vi "PRISM_RasterScan_BSC202(T-Dimension_Added).vi"() -> ()   [LabVIEW 2022 SP3]
uses:
  C:/Users/ulate/Documents/mnOP/mnOPSuite-main/PRISM/Thorlabs.MotionControl.Controls.dll
  mnOPSuite-main/PRISM/Thorlabs.MotionControl.Controls.dll
  C:/Users/ulate/Documents/mnOP/mnOPSuite-main/PRISM/Thorlabs.MotionControl.KCube.StepperMotorCLI.dll
  mnOPSuite-main/PRISM/Thorlabs.MotionControl.KCube.StepperMotorCLI.dll
  <vilib>/Analysis/NI_AALBase.lvlib
  <vilib>/Analysis/baseanly.llb/Mean (DBL).vi
  C:/Users/ulate/Documents/mnOP/mnOPSuite-main/PRISM/Thorlabs.MotionControl.Benchtop.StepperMotorCLI.dll
  mnOPSuite-main/PRISM/Thorlabs.MotionControl.Benchtop.StepperMotorCLI.dll
  mnOPSuite-main/PRISM/Control_PRISMRasterScan_ActivityLoop.ctl
  mnOPSuite-main/PRISM/Control_LineScanCounterAE.ctl
  mnOPSuite-main/PRISM/Control_PRISMRasterScan_ProtocolsLoop.ctl
  ActionEngineEnum.ctl
panel:
  in  "t Action":T1=enum."Done"
  out "t - Current Position (mm)":dbl
  in  "t Motor Settings":T2={"Step Size (mm)"=10.0, "Initial Position"=0.0, "Move Absolute/Relative Position"=0.0, "Step Delay (ms)"=0, "Velocity (mm/s)"=1.5, "Acceleration (mm/s^2)"=1.0} {"Step Size (mm)" min=0.00046 format="%.8f"}
  out "t error out":errorcluster
  in  "KCubeStepperControl t":refnum<k24>(container)
  in  "SerialNumber t":string="26004283"
  in  "Update origin":bool
  out "Protocol status":string="Ready for protocol!"
  in  "Protocols":T3(tab)=enum."Saved Positions"
  in  "Target coordinate":T4={"X coord (mm)"=13.679193173363094, "Y coord (mm)"=17.37439041210012, "Z coord (mm)"=19.037080609490427, "t coord (mm)"=0.0}
  in  "Move to target":bool
  out "Origin coordinate":T4={"X coord (mm)"=13.208955078125, "Y coord (mm)"=17.107802734375, "Z coord (mm)"=19.036842575356477, "t coord (mm)"=0.0}
  in  "Update target":bool
  in  "Move to origin":bool
  in  "Stored positions":T5(array[cluster])=[{"X coord (mm)"=15.5859716796875, "Y coord (mm)"=15.71225830078125, "Z coord (mm)"=19.053150660079638, "t coord (mm)"=0.0}, {"X coord (mm)"=13.679193173363094, "Y coord (mm)"=17.37439041210012, "Z coord (mm)"=19.037080609490427, "t coord (mm)"=0.0}, {"X coord (mm)"=9.08337158203125, "Y coord (mm)"=16.38648681640625, "Z coord (mm)"=19.027052048324006, "t coord (mm)"=0.0}]
  in  "Stored position names":string[](array[string])=["Gold", "Corner", "Shane region"]
  in  "Move to\nstored position":bool[](array[boolean])=[FALSE, FALSE, FALSE]
  in  "Store target\nposition to":bool[](array[boolean])=[FALSE, FALSE, FALSE]
  in  "Do Linescan":bool
  in  "Linescan points\n(relative x,y, microns)":dbl[][](array[numeric])=[[134.75975910445754, 60.57194852467012], [148.27256923926274, 62.20847306409274], [161.7853793740679, 63.84499760351537], [175.29818950887307, 65.48152214293799], [188.81099964367826, 67.11804668236061], [202.32380977848345, 68.75457122178324], [215.83661991328862, 70.39109576120586], [229.34943004809378, 72.02762030062848], [242.86224018289897, 73.66414484005111], [256.37505031770417, 75.30066937947373], [269.88786045250936, 76.93719391889636], [283.4006705873145, 78.57371845831898], [296.9134807221197, 80.2102429977416], [310.4262908569249, 81.84676753716423], [323.93910099173, 83.48329207658685], [337.4519111265352, 85.11981661600947], [350.9647212613404, 86.7563411554321], [364.4775313961456, 88.39286569485472], [377.9903415309508, 90.02939023427734], [391.5031516657559, 91.66591477369997]]
  in  "Linescan Accumulations":i32=11 min=1
  out "Current point":i32
  in  "Halt linescan":bool
  out "Current\naccumulation":i32=11
  in  "Generate\n# points\n(cursors 1&2)":bool
  in  "# Points":i32=20 min=2 max=100
  out "X stepper reference":refnum<k24>
  out "Y stepper reference":refnum<k24>
  in  "BenchtopStepperControl Y":refnum<k24>(container)
  in  "BenchtopStepperControl X":refnum<k24>(container)
  in  "Save Image":bool
  in  "Path to save image":path=path "D:/Dropbox/Data/PRISM/2023.05.23 - Brayden - CalibrationExperiment - 119nmGrating/5x5_9.1micron_monochromated.txt"
  in  "Move to cursor 1":bool
  in  "Auto-level phase":bool
  in  "Acquire":bool=TRUE
  in  "Settle Time Y":u32=500
  in  "2nd sideband factor":dbl=1.0
  in  "Settle Time X":u32=50
  in  "Py":dbl=-38.62030580980725 format="%_3f"
  in  "Px":dbl=63.19603906604226 format="%_3f"
  in  "1st sideband offset":dbl
  in  "Phase offset":dbl=-7.0317445278654365 format="%_3f"
  out "Phase":dbl[][](graph)=[[-0.022387540499821057, -2.058073888022488, -2.674115903484436, -2.9544519791983532, 0.9804648819298123, -0.21571753535931215, -1.8423350309242874, 1.9906478539609171, 2.5360374269275248, 2.656112089306447, 2.35744039612554, 1.9479416381106667, 1.3283110045095121, 0.8287830160341692, 0.0015003367418202629, -0.6042101212176902, -1.313129505955537, -2.0121744959565113, -2.8202574981697097, 2.82386999642312, 2.1056236578858005, 1.3825868635958933, 0.6516979802989589, -0.11705277330859332, -0.8663526332155058, -1.6488935896277255, -2.3898283311918362, -3.111747881862428, 2.354022610449217, 1.5981909201102198, 0.999097752100301, 0.11666767544505063, -0.6255420967363605, -1.344064191404911, -2.1083959373327517, -2.8419430799594565, 2.667384503490176, 1.9637011456735003, 1.2230875404057322, 0.49976096613480436, -0.19396741539229012, -1.0079793141447588, -1.7125457563331672, 3.059263850520008, 2.2710943441974045, 1.4829248378748154, 0.6947553315522121, -0.09341417477039116, -0.8815836810929802, -1.6697531874155693], [1.3628880674624408, -0.2630817845670128, -0.10980599380193556, -1.8345316004921504, -2.204085976347738, -0.14179729710883748, -1.2847852512940126, 2.9634721346216164, -2.815473176799607, -2.5973907021062708, -2.922850019605578, 2.9635213410531325, 2.4514727389564435, 1.8030287953244226, 1.0294730194139348, 0.4576671275139077, -0.27089481789525394, -0.9873673943323595, -1.7804895356639534, -2.3687185763918244, 3.14003843880214, 2.318275957039088, 1.737089720416126, 0.9172648738715132, -0.21566467221115104, -0.43893815331455244, -1.326304504354333, -2.0795219597874492, -2.916987708315201, 2.695457261994612, 2.0229011483410417, 1.171918489139145, 0.43802228817759925, -0.2801368330695517, -1.0396590157832648, -1.8024496700734431, -2.5632904960467613, 3.040122676411002, 2.346330734522372, 1.5444701977180024, 0.8263618586431427, 0.05569318859598482, -0.7071801917261205, -1.9342063736791282, -2.7223758800017315, 2.7726399208552657, 1.9844704145326624, 1.196300908210059, 0.40813140188747, -0.3800381044351191], [-3.066884103109013, 0.9729599729543059, 0.8274657505887806, -0.8521734837812724, -1.7610376922341295, 1.5856394803568339, 0.1268857548291482, -1.9691799992391434, -1.4484367584059132, -1.2676123760144762, -1.6187348635530725, -2.0480064271227203, -2.4007798568858334, 3.1161499915202935, 2.3473474349846413, 1.7619068509469216, 1.0789468726915707, 0.37216732621407544, -0.4886782343943743, -1.0358510858881864, -1.7925323857931978, -2.602999261436789, 2.9510587581194585, 2.2525199600469996, 1.2937303676530512, 0.8952483171540173, 0.010397577352765808, -0.704939673587532, -1.6342691150966857, -2.218708036019933, -2.9599800502081486, 2.5159200741562735, 1.8299109061018193, 1.0253986988047359, 0.25924289190646377, -0.49860314852613996, -1.2596561474008254, -1.9321767682116544, -2.6680856525186627, 2.866214678319018, 2.2123793056056122, 1.3704893856878222, 0.6060059677024476, -0.6444912906986779, -1.432660797021267, -2.2208303033438703, -3.0089998096664594, 2.4860159911905235, 1.6978464848679202, 0.9096769785453311], [-2.3965980652031176, 1.6227568075408518, 1.168964897317034, 1.4095316197290177, -2.8014709215206857, -2.2329707988617766, 2.1851936633849363, -0.34485343356651654, 0.14279525512465874, 0.3540126356171065, -0.044315893155403074, -0.482972843851039, -1.002422538441758, -1.6853905594341434, -2.440464573629015, -2.8891213399429176, 2.5877374062332876, 1.8374526951417636, 1.1486396741771507, 0.5247186443110969, -0.26949674326147743, -1.0848567982945525, -1.848210887792014, -2.5387805815220865, 3.0687085163085435, 2.3387104464322164, 1.54582113363902, 0.8121802971552299, -0.03824350311151292, -0.6778476179916666, -1.4224225887198862, -2.229314349052679, -2.944827148116417, 2.5193975756285525, 1.8168759345426118, 1.0311792634079424, 0.29301642014190676, -0.46532133283141874, -1.0983502953965996, -1.9054318285761838, -2.5634056945953745, 2.9290667229416556, 2.1510820393184567, 0.6452237922817723, -0.1429457140408168, -0.9311152203634201, -1.7192847266860092, -2.5074542330086125, 2.9875615678483705, 2.1993920615257814], [-1.6841800797532274, 1.81433573403317, 1.9335449128509756, 1.4953972828545172, -1.608539055796733, -0.7086282362391554, -2.492175019225904, 1.1043658709546023, 1.6255459898063904, 1.7377721010176739, 1.4066056895155938, 0.9893110706463943, 0.41623260003367335, -0.42402667241574044, -1.0364775587393407, -1.5391521320349355, -2.4206609441522122, -3.097728525000063, 2.5361868143635213, 1.9845966715424126, 1.1191387411501275, 0.24604967911620435, -0.4740298321180312, -1.2495097740212167, -1.8317788479276942, -2.5951763567334396, 2.937298895851523, 2.2443865176780733, 1.3180121470375852, 0.5932561040055369, -0.03891982944377759, -0.8281018784912177, -1.4177150586273903, -2.2919076513566807, -3.069067654983254, 2.446145320515516, 1.7009132945316843, 0.8706102384085312, 0.2977063161632074, -0.4803340445821007, -1.1888387915909675, -1.9456314651204565, -2.84988979467969, 1.9349388752622367, 1.1467693689396334, 0.35859986261704435, -0.42956964370555895, -1.2177391500281622, -2.0059086563507513, -2.7940781626733404], [-0.8973343669603029, 2.123126138782993, 2.8199224507415517, 1.905484194967828, -1.127661496481934, 1.174155302549254, -0.8533196886458425, 2.6598834334499006, 3.075510546275801, -3.10785068992406, 2.7955257385388705, 2.412595201150511, 1.8555829163744129, 1.1888865219585476, 0.5176127773060646, -0.1418990848609507, -0.920191338355826, -1.5600168316567231, -2.293106731159032, -2.836949357060698, 2.5281579597586266, 1.8007761476738473, 1.0855407276800229, 0.27144007547231297, -0.36334755803092733, -1.1714381725212952, -1.9216266601785001, -2.6465573895732213, 2.8876005318127866, 2.1127905891614738, 1.3791718764432055, 0.5015637852025137, -0.08529276139088182, -0.8980377283577994, -1.672430623348692, -2.3824589331447292, 3.104730299921389, 2.4645905880971313, 1.72661821951014, 0.922796133288017, 0.19702009512686658, -0.5421983101135623, -1.2888533901549053, -3.058531348936903, 2.436484451920098, 1.6483149455974946, 0.8601454392749055, 0.0719759329523022, -0.7161935733703011, -1.5043630796928902], [0.08388963387707804, 2.906088721948243, 2.6850986349242767, 0.27512112222713636, 1.1091449624488927, 2.5073112355343996, 0.7899138334549409, -2.1604437613067216, -1.811580954875117, -1.7532620930163745, -2.0518609798455962, -2.406820073200329, -2.9886310634991364, 2.6116717182552023, 1.8510266765310348, 1.2843187293208533, 0.4296141672480793, -0.22785376121727374, -0.9773335792860802, -1.492074426042434, -2.33843645279439, 3.126300272992971, 2.3987147516140475, 1.592480069562761, 1.0353996771496732, 0.21793488873515088, -0.4725206147675465, -1.2331384498445779, -2.052011387265793, -2.7718324467228115, 2.8171907769568136, 2.0922645338624832, 1.2879170715464276, 0.43866550742682264, -0.27113986038910554, -0.9592680085289338, -1.785050188935319, -2.344856830069869, -3.124976762825561, 2.3015383661274385, 1.666433266139851, 0.8354098135605348, 0.12994388903859644, -1.7688162659564455, -2.5569857722790417, 2.9380300285779484, 2.1498605222553557, 1.3616910159327524, 0.5735215096101491, -0.21464799671243995], [0.7730064791060114, -2.2422916004447355, -2.7603924915974503, 2.43347466633578, 0.08731074224383217, -2.308316997016306, 2.393768121573377, -0.7118451463719238, -0.3355634717218221, -0.341494301675878, -0.6173869601886164, -1.024429550421761, -1.6166729606095078, -2.2341935145882683, -2.911480529054126, 2.7224483054582116, 1.981053415771921, 1.2218363391617988, 0.6523104836249072, -0.059507404315208845, -0.9535593178525446, -1.6193221075455906, -2.3700117432027543, -3.1250855773976536, 2.4788625057042744, 1.5463840538120408, 0.9800371354102033, 0.19579475094657184, -0.5653468704770397, -1.3707899976227438, -2.052383065739953, -2.789031304527679, 2.713926729646005, 1.8692635741312635, 1.1709183504774643, 0.45359994241800194, -0.3443418710311015, -0.9802643856205293, -1.765450941430231, -2.581249237757593, 3.043986042708198, 2.265111288961471, 1.5420804523152292, -0.47910118297598814, -1.2672706892985843, -2.0554401956211805, -2.8436097019437767, 2.651406098913206, 1.8632365925906136, 1.0750670862680245], [0.2580695237139876, 0.6828682232009009, -2.0469861827754645, 2.946288830382736, 0.6935475619157456, -0.10756103977141507, -2.2857382865566542, 0.712782643772337, 1.1093310428349588, 1.1774677065998338, 0.7947546112530475, 0.3567449711397579, -0.2272672897086636, -0.7640476232136955, -1.5475436693311009, -2.148207546509873, -2.8732833743547275, 2.614759429965167, 1.9901999575950011, 1.3305097400488837, 0.155054665233056, -0.2799398459732281, -1.129929015531875, -1.7955541373238404, -2.3900822532263497, 3.0472113011399973, 2.3715703347198698, 1.6539055221121153, 0.7409813253426805, 0.07315321432771427, -0.6342971726609861, -1.3299365984528642, -2.0538581044309687, -2.916252721124213, 2.5622245639023866, 1.8576744350770582, 1.068926198989402, 0.4247753644850647, -0.37687037047335536, -1.1670272987173398, -1.7851786584145728, -2.603830732259585, 2.904408054135054, 0.8106139000044621, 0.022444393681865904, -0.7657251126407303, -1.5538946189633265, -2.3420641252859298, -3.130233631608526, 2.3647821692484747], [-3.115997453644919, 1.3909049739370483, -1.9508788518699776, -2.9830523341856505, 1.6363109571985834, 1.2173345121005736, -0.739468648264018, 2.103685643131244, 2.5505355075887337, 2.5707732107446466, 2.268128255213327, 1.7210402472322528, 1.2308655811346911, 0.6085752294328506, -0.1483003340097877, -0.7464704859366584, -1.4736619725918327, -2.132855638872755, -2.9063750039330003, 2.728870665982347, 2.2285459060256656, 1.2752214884418969, 0.40971309866165306, -0.2857114181179359, -0.9826548217669391, -1.8061567137429009, -2.4775345698111977, 2.9629138369751384, 2.2654765680432583, 1.507411181145983, 0.7777850501704258, 0.07485373885175406, -0.6578077982824837, -1.4464199927970682, -2.2489490333640596, -2.981886614680178, 2.4773857903899454, 1.8533544801102124, 1.0099960800319217, 0.25794269886597476, -0.38849009668585666, -1.163266010818134, -1.961255983791105, 2.1003289829849194, 1.3121594766623232, 0.523989970339727, -0.26417953598286914, -1.0523490423054724, -1.8405185486280686, -2.6286880549506577], [-2.973824639667331, -0.3808371761856719, -1.2697167652686812, -2.250656583574277, 2.8690963540737027, 2.8392143717039797, 0.8135335245491242, -2.709993525842972, -2.3106513014105543, -2.3472060220939985, -2.5575537636549854, 3.120687882907709, 2.6305678861935364, 2.0085906949027024, 1.2420061608844648, 0.6335744611619436, -0.09758461693938791, -0.7620617457308008, -1.4573633096672136, -2.1472818673513068, -2.9396884225341697, 2.611867804818674, 1.738198702707928, 1.017938761103924, 0.40206618714671905, -0.3647565931770451, -1.1125631607993025, -1.829479741397277, -2.6132072700993483, 2.939980242492741, 2.1431631699713876, 1.4903147682332616, 0.7395956791538545, -0.09560326657526019, -0.8023186722421976, -1.55563412134617, -2.3724378835270095, -3.034613022697915, 2.4875320249892674, 1.7179354468544759, 1.0208687081664785, 0.2498819015875675, -0.5050262473460911, -2.8931412412142166, 2.6018745596427735, 1.8137050533201773, 1.025535546997581, 0.2373660406749778, -0.5508034656476184, -1.3389729719702075], [0.5200492600706852, 1.2630973959723146, -0.4740267800265876, -0.7403538003570418, -1.6536060683733167, -2.0800365358772215, 2.4503654239413013, -1.2585126799975002, -0.8877822370387727, -0.9313533566473948, -1.1973711148108261, -1.7177401303750703, -2.2263558951525066, -2.874595724811934, 2.643689238760323, 2.073831528075572, 1.3301628193342507, 0.6522957131674332, -0.03622715939361232, -0.7544934399100285, -1.5390794884192118, -2.17326521527799, -2.999659231466655, 2.4617200925048355, 1.7929092616516815, 1.072060080063185, 0.29209005208340777, -0.39856959907451994, -1.211737276911128, -1.8932740737540161, -2.7594350636974756, 2.8818784687951045, 2.1116870898451943, 1.3089986080179088, 0.5857604140665451, -0.12920431168853597, -0.9877530526656138, -1.6554457047385895, -2.297444796234501, -3.136121230809234, 2.4431058249097504, 1.6399261598454018, 0.8980115659296111, -1.6034261582337592, -2.3915956645563554, 3.1034201363006346, 2.3152506299780384, 1.5270811236554351, 0.7389116173328389, -0.04925788898975014], [2.63144226038483, 0.9159796062842211, 0.8148153720736673, 2.2229748004338425, 1.6597418954745944, 0.12500012644730596, -2.188188428011288, 0.12953008990672243, 0.5354117393527269, 0.5605386086139181, 0.27220915667070233, -0.32470787147026137, -0.8245857182912424, -1.4125876806890567, -2.162082774030769, -2.7861030461041087, 2.741577123264112, 2.064156988818894, 1.350300620866169, 0.6459662428196582, -0.1368522323671515, -0.7598783694100684, -1.7426266871290785, -2.494107127160623, -3.0597182984750315, 2.4897416285507266, 1.721901121176444, 0.978720137474582, 0.2104638963564689, -0.5237560149787885, -1.265032459304063, -1.9667583670298985, -2.5608275456716996, 2.7380715771498245, 1.9862497902215175, 1.2249432166041636, 0.4281864726916531, -0.26963311237808085, -0.9325424554760424, -1.7122382135179528, -2.3807662581600653, 3.0389706582874076, 2.3369497205983585, -0.31371107525330544, -1.1018805815759016, -1.8900500878984978, -2.678219594221094, 2.816796206635889, 2.0286267003132927, 1.2404571939907036], [-2.173046144746042, 2.327754642837995, 2.0167744248018664, -1.599981212059376, 2.4319056703568442, 2.0462184480633585, -0.6718391581152456, 1.644926193302597, 1.9837125530979485, 1.982008320024092, 1.6609081524153577, 1.0857671008069953, 0.5869947955236339, 0.004662963761767003, -0.7233032604903449, -1.3813132647547528, -2.1145798550152133, -2.7747600031149076, 2.7343741359794933, 2.073926005058061, 1.2764889784333215, 0.6533578407238547, -0.17102646990525017, -0.8929948778087553, -1.548835399495994, -2.439305784995627, -3.1345435928506955, 2.3825028990283688, 1.6455912716073495, 0.8527094940419708, 0.19601914159793843, -0.572055528303034, -1.3646559548139052, -2.1223782739691828, -2.85986707440755, 2.60045574960424, 1.8911951423258344, 1.1223577581701818, 0.5584264226813822, -0.3071117581792997, -0.9733969407070333, -1.835276479165696, -2.5351578867511115, 0.9760040077271483, 0.18783450140455216, -0.600335004918044, -1.3885045112406402, -2.1766740175632435, -2.9648435238858397, 2.5301722769711574], [-2.884860960819294, -1.7513434146345777, 0.7123014767375171, 0.1943540711077354, -2.5385134853657014, -2.699555026183873, 0.7646123564405336, 3.0923353048496853, -2.869915989855963, -2.8195292937797305, 3.040276995153012, 2.5347839323059045, 2.025477092586182, 1.429012362057347, 0.7390922961161026, 0.028608660927178065, -0.726673509444641, -1.432249952329133, -2.127407817223622, -2.792821541195755, 2.7983619838585234, 2.074199666133242, 1.138201779148008, 0.3989645280389098, -0.1399267438708902, -1.0559672393774004, -1.670301430922831, -2.502388981537454, 3.058322333465547, 2.250496525707705, 1.5784245972928943, 0.8344382636910481, 0.07549979434488918, -0.7460982483501208, -1.4478775376463684, -2.1835461868862076, -3.0046115905035045, 2.5810028674209065, 1.9384457724066628, 1.1263868485807684, 0.39669676090830563, -0.3870139460729902, -1.1604800445496366, 2.2657190907076057, 1.4775495843850095, 0.6893800780624133, -0.09878942826018289, -0.8869589345827862, -1.6751284409053824, -2.4632979472279715], [-0.7852097056049878, 2.1081468430841728, 2.7945248660693203, 1.892666528646492, -1.346574954754363, -1.1578876479767892, 2.196206649700404, -1.8529822833943292, -1.5252907241381832, -1.363214299505291, -1.8320123881653716, -2.3675057234843866, -2.8730168807639984, 2.837429048956743, 2.1330312818233166, 1.4491870262157747, 0.6886986436454521, 0.028034348044742696, -0.6824241972907128, -1.3214913370120585, -2.129124822209228, -2.75152449060268, 2.6711262282632093, 1.9919669751615992, 1.1729537755615542, 0.41281981259588285, -0.30177477381469053, -1.0291253323000777, -1.8268347278026624, -2.5841575004119512, 2.9760980651843134, 2.271142398497169, 1.5303077805668455, 0.6851942217339246, -0.06638121104411887, -0.7559505870880336, -1.6073697794968247, -2.2972219446696354, -2.9241144647628605, 2.604725648945948, 1.8210503364421413, 1.1173064118856892, 0.24947788648885094, -2.7277511334915303, 2.7672646673654597, 1.9790951610428635, 1.1909256547202673, 0.40275614839766405, -0.38541335792493214, -1.1735828642475212], [-2.709526966188239, -0.3812157791770616, -0.12614908608763642, 1.2006492434692362, -0.825491872620816, 0.49124666558333985, -2.553079815155952, -0.3937757240518831, -0.088966679885365, -0.009173515307265845, -0.4141906935124364, -0.992320504738121, -1.4418907098008527, -2.0067230057162035, -2.7198045957605146, 2.8305454061780395, 2.0761699938474782, 1.442218255494307, 0.7866714072604735, 0.09716927015514987, -0.7309537991380184, -1.3346666278509205, -2.236571642604603, -2.987519409350255, 2.5353584232900577, 1.7898752666074849, 1.069774142818023, 0.3549653122171632, -0.39106485113418454, -1.142079815317187, -1.8729632219726273, -2.5783700432487677, 2.8654644364564845, 2.1411552498367357, 1.3123252465222315, 0.6374832018004728, -0.16938779360920186, -0.8238032985401098, -1.537513755821685, -2.27126609535015, -3.0334470118370724, 2.5710513376407995, 1.7029453791897282, -1.438036050511073, -2.226205556833669, -3.0143750631562654, 2.4806407377007247, 1.6924712313781214, 0.9043017250555252, 0.11613221873293611], [-0.6698893459784507, 2.224757190115138, -1.929418603559423, 1.3527360891611764, 0.05830593398933992, 1.9802343533654074, -1.0026363986646487, 1.0998302513821905, 1.3892978745956555, 1.3734377812975787, 1.059816044743254, 0.4615306076974548, 0.0011970642299843348, -0.5956531889249419, -1.2634306478415276, -2.0239544459616656, -2.8305840324069393, 2.8772258502850283, 2.229552032212803, 1.4849068332061561, 0.676538937259922, 0.08913797767668719, -0.7565036347874026, -1.435366700771486, -2.3363085433156154, -3.062663537832218, 2.5087316407522957, 1.800965273555053, 1.064523403406172, 0.2866122181004407, -0.5365823710689348, -1.129169618801594, -1.9670985496325883, -2.7301287774478453, 2.8271880473914397, 2.049980367992461, 1.2869164057899454, 0.5841585935737381, -0.16667141215573977, -0.8464015288862576, -1.6400130135771374, -2.379895952818176, 3.127334169829446, -0.14832096753062274, -0.9364904738532189, -1.7246599801758151, -2.5128294864984113, 2.9821863143585716, 2.1940168080359754, 1.4058473017133863], [2.178696134477395, -1.0546034523203751, 2.4884070790795256, 2.123437245090617, 1.835263556075617, -2.4977562500992967, 0.6493906510835998, 2.489636111468748, 2.8509749648899714, 2.750640944385882, 2.441422455515454, 1.948380988121169, 1.413904060409216, 0.9063075384573587, 0.09345992313698481, -0.6293282595949794, -1.348722072853203, -1.9440713596479178, -2.623998442502777, 2.9020028912852602, 2.078070242797306, 1.464674289431886, 0.6812573499239227, -0.13355103892651998, -0.8916037174405327, -1.5645054582399482, -2.3119385078920165, -3.088379875058524, 2.5058119196160495, 1.7310830201055616, 0.8851984054452169, 0.26463137336722653, -0.5171885246636911, -1.3337743686308254, -2.130881604317665, -2.8248107654453705, 2.667910485189738, 1.9870789935094066, 1.3041041622715959, 0.5516458662809818, -0.21644390353997345, -0.9772662807632528, -1.7404750072504367, 1.1413941154498346, 0.3532246091272384, -0.4349448971953578, -1.223114403517954, -2.0112839098405573, -2.7994534161631535, 2.6955623846938437], [-1.8287562708843872, 0.04768632953219765, -2.467116732188604, -0.03391991924946325, -2.413205599950466, -0.8094068070543177, 2.2403086150990354, -2.317858274410181, -1.9992759356323901, -2.088217448326489, -2.4467709689218555, -2.976173025207144, 2.85903492302813, 2.280349601733013, 1.5288108026358849, 0.8167115205507365, 0.13126729408893922, -0.49440091737684355, -1.170913713785266, -1.9557726210624917, -2.767154323505766, 2.834087862542571, 2.2398033094130003, 1.3491982644127907, 0.5476037466268222, -0.22082665184621986, -0.9005498972498964, -1.6438696712077796, -2.332060577662606, 3.109825824257781, 2.3457121107665726, 1.6302596069984423, 0.8791727717174318, 0.1657119878403126, -0.5562678267205889, -1.3970085208570104, -2.2165776350130386, -2.893300276842215, 2.665140649782643, 1.9577808270846297, 1.2096961512692044, 0.4176585999306681, -0.3179688499827371, 2.431109198430285, 1.6429396921076886, 0.8547701857850925, 0.06660067946249626, -0.721568826860107, -1.5097383331827032, -2.2979078395052923], [-0.7683439806474119, 0.7501439736611388, -1.550617798286094, 1.0493661311339118, -1.1686758043916683, 0.7903291994174424, -2.5226564786612116, -0.9546125833302632, -0.5470890635774577, -0.6525023602947719, -1.0294153618979003, -1.5668225325855065, -2.0540698470964944, -2.6596544404939486, 2.925825891431856, 2.1976701755388834, 1.5558480442451632, 0.8988477385385867, 0.21539576132037652, -0.557730163409218, -1.2920222871051674, -1.9595815458115515, -2.71145655451648, 2.619823145581641, 1.9722792462605003, 1.246399029920779, 0.4954495306730595, -0.2098103687168993, -1.0071181399987443, -1.7475341709055203, -2.5343971502553644, 3.0983937971391615, 2.2990498738479204, 1.5241985230404502, 0.8301007793357638, -0.007043439218509029, -0.7962645098185046, -1.4884174929052278, -2.132021930330863, -2.957563821971398, 2.6154601248937013, 1.9404595416098758, 1.1096473383198369, -2.562361025768844, 2.932654775088146, 2.14448526876555, 1.3563157624429536, 0.5681462561203503, -0.2200232502022459, -1.008192756524835], [-0.5327729173084137, 1.1817186868805862, -0.5244973747871988, -1.2439217995780396, -0.8892931005313613, 2.4515388617475757, -1.062850907130148, 0.5103538414739681, 0.8156232332962041, 0.843693781783525, 0.3336130049808297, -0.1027437313835815, -0.6699768759071443, -1.2628240914782918, -1.9076765568238603, -2.7260101600313966, 2.960500823970566, 2.3286897369519775, 1.6018707630370947, 0.8057410248164967, 0.1055475440001068, -0.5612677425767636, -1.3154802434523258, -2.041041668967254, -2.9606055255255486, 2.59606161656081, 1.8917725623469162, 1.1562058060421059, 0.3884617615694044, -0.2639263799211551, -1.1709663361525182, -1.7483886878074202, -2.552001555054612, 2.9141239196991613, 2.210711768338352, 1.3983237589437563, 0.6506860617403785, -0.11842622680805626, -0.7660539543327332, -1.6115292214871157, -2.259522565069391, -2.9479360580366887, 2.4970164979595673, -1.2726459427883867, -2.060815449110983, -2.848984955433579, 2.646030845423411, 1.8578613391008076, 1.0696918327782114, 0.28152232645562236], [-0.0023691169747195318, 2.2405029639283462, -1.4136789713513274, -0.3873187850142905, 1.7329829857476362, -2.2813584855433717, 0.47090808812390605, 2.0419903622176783, 2.238498055681031, 2.195299612484366, 1.7647394464191244, 1.3163166111065294, 0.7837364642034714, 0.1192873134390009, -0.45725297449630276, -1.316068276434855, -1.8706007613256848, -2.5240876041224123, 3.028499211149768, 2.212481410723255, 1.5232244265175687, 0.8338055061011751, 0.10286740803684147, -0.6852887494162552, -1.5658450738416283, -2.2445825094163183, -2.929259174655508, 2.5572152595775695, 1.7937195353712658, 1.0937577867868296, 0.2407320435286393, -0.3659477328164482, -1.2162657707361348, -1.972344243676242, -2.675581448053344, 2.809296069567192, 2.0864698214763457, 1.2861361227177728, 0.665833564279267, -0.20407620829174533, -0.8774968336975126, -1.63400466819372, -2.355711743080608, 0.017069140192063514, -0.7711003661305327, -1.5592698724531289, -2.347439378775725, -3.1356088850983284, 2.3594069157586617, 1.5712374094360726], [2.3377656726954363, -2.4258935878055965, 1.7421573971991613, 1.091667428381598, -0.2770355796014563, -0.8273713422296538, 2.013751590415456, -2.8111194080978734, -2.5185943120435894, -2.6896908726807034, -3.0767848791952552, 2.753109268910105, 2.1984191767330437, 1.494091244012278, 0.9470765049590888, 0.12385435033179348, -0.42240436998485364, -1.133550248196869, -1.8798630493253334, -2.5964236733560977, 2.9272337678842426, 2.2569657556867817, 1.4712641647999227, 0.7158144479370527, -0.1593222306805604, -0.8829409742027892, -1.5137783149943242, -2.3420103873077522, -3.071013267117758, 2.42612212245894, 1.6888831235999024, 1.05217369030475, 0.16016851788712572, -0.5947600895818028, -1.291972990162935, -2.035259636501891, -2.7842114344197846, 2.710146097261017, 1.9970582564600612, 1.2301137022641413, 0.6258173156845253, -0.29209911764016105, -0.9741102311721814, 1.3067842231725209, 0.5186147168499247, -0.26955478947267153, -1.0577242957952677, -1.845893802117871, -2.634063308440467, 2.86095249241653], [-2.4506858922883907, -1.379630401264695, 2.778622610171844, 3.0334974454987247, 1.2075029888122693, 0.726676996063965, -2.726274859081876, -1.3386576818314992, -1.097780399012283, -1.2480625547482376, -1.6054051701564447, -2.10519432589145, -2.650034301266391, 2.8766643012695567, 2.3353383762853177, 1.4568273904801394, 0.8589336973397614, 0.2547028525392818, -0.48377900141125885, -1.2073515723525006, -1.955986065604499, -2.611848727614751, 2.9117999172020568, 2.0755341291204203, 1.3127814052719255, 0.5826805037430614, -0.16150628622354546, -0.9271413601570231, -1.67129705461066, -2.4529797995758607, 3.098506180963799, 2.4060014469171414, 1.5653551069965115, 0.8059859758229493, 0.03961726734288096, -0.6365130485621657, -1.3881025063145986, -2.1445934354764766, -2.8255762666750996, 2.7093576063539437, 2.0121447644944688, 1.1092470876937366, 0.3935716374311049, 2.596499306152971, 1.808329799830375, 1.0201602935077787, 0.2319907871851825, -0.5561787191374208, -1.344348225460017, -2.132517731782606], [-1.532776907052778, -1.3092675650156345, -2.978369736370965, -2.432150051129259, 1.966318508425644, 2.3426407860243224, -1.2288596062969397, 0.05238858697865467, 0.27866636585380533, 0.19906908729653594, -0.17774744560040645, -0.684472374246873, -1.27245396756339, -2.0179025693023434, -2.5755680557616394, 2.955552653382984, 2.2451907169525533, 1.6368425894938703, 0.9217328466995305, 0.14911722908330738, -0.5221142802212491, -1.2197332899442141, -1.9591799406385348, -2.7426511700515164, 2.694035725398299, 2.018935016749694, 1.2190956398746078, 0.48560306285228805, -0.2903744591731332, -1.0551366946040872, -1.777068887977455, -2.462577164106368, 3.0220189513587012, 2.233440688812049, 1.3824057640448366, 0.743166806113261, -0.01367967497327971, -0.7216881250005516, -1.4570577903354316, -2.1276894776076993, -2.936650623186912, 2.5266895893518093, 1.7585657923718916, -2.396970918046158, 3.0980448828108322, 2.309875376488236, 1.5217058701656399, 0.7335363638430366, -0.05463314247955964, -0.8428026488021487], [1.2428508538451304, -1.3951202562568419, -1.7349104376200941, -1.4578966380928478, -2.7382853282641655, -2.1820108196442334, 0.279534148781611, 1.4847920035644755, 1.7217396757664538, 1.607772481666359, 1.2210688701900878, 0.731970627929261, 0.08917626304189952, -0.5179691108910376, -1.1943297180021446, -1.8263818156258473, -2.571211358487684, 2.9741001797960287, 2.294537358957353, 1.579492639947052, 0.8505819734683442, 0.12325830552093109, -0.5378873799685593, -1.3485517940570624, -2.190665846186036, -2.965261513940252, 2.6452466967513626, 1.8948330229005474, 1.125916814912502, 0.36897182108414484, -0.3865598295876129, -1.1031515606397129, -1.8637714324613466, -2.6266086141790765, 2.810013793307398, 2.1100663288559325, 1.3263763620717155, 0.6908860050040282, -0.040216309110186366, -0.8457455451422504, -1.5514788554081118, -2.2694661765435775, -3.086618043367725, -1.1072558350657076, -1.8954253413883038, -2.6835948477109, 2.81142095314609, 2.023251446823487, 1.2350819405008906, 0.4469124341783015], [1.1250431941262384, -3.0203364938122483, -0.8590960672811327, -0.5205494764362157, -1.956494144306891, -0.4217940909064808, 1.7177812820167482, 2.944307653662694, -3.138977268649544, 3.0591232558639128, 2.6990150410400737, 2.128633782669823, 1.5341679904956464, 0.9320963249651868, 0.2301405625160129, -0.40214491970724353, -1.151014075689364, -1.8817059444177424, -2.5850417636785394, 2.9620322305325715, 2.1591320247291783, 1.506601919153649, 0.8474605159652704, 0.09714820951370662, -0.7250065085151114, -1.4844874612268057, -2.2203660783267587, -2.984669099311864, 2.4953605383740562, 1.8007197467309588, 0.9912374523719798, 0.24590027277474347, -0.4925968243475678, -1.2902543714923156, -2.062155710429759, -2.821971508725537, 2.6884633276288046, 2.091015420033356, 1.3618600367828364, 0.5985716068395996, -0.2035811188070955, -0.8836474038163615, -1.6514257443272538, 0.18245924791474977, -0.6057102584078464, -1.3938797647304426, -2.182049271053039, -2.970218777375642, 2.524797023481348, 1.7366275171587588], [1.238976688546142, 3.0748379058144657, 0.08291986112693195, 0.63637126425375, -0.08045209310738244, 1.1302307493406794, -3.121955089503846, -1.919689818885768, -1.6983212017830347, -1.8538503691081054, -2.1319491304693194, -2.7472480449297585, 2.9641510621526734, 2.28458785864251, 1.6407242629808074, 0.9598020979147925, 0.27146438099768133, -0.42319817494381695, -1.192418885849765, -1.9025339926327725, -2.6442222363854277, 2.938658538403139, 2.1967688930728038, 1.4671244326300474, 0.6532987532659398, -0.145274704839089, -0.8270665527127719, -1.603088381060589, -2.35333088767288, -3.123602137914668, 2.370246347964226, 1.7308499364785792, 0.9095877496945928, 0.06491193204418444, -0.635419128328548, -1.3663121866938406, -2.160488718252274, -2.8381501265457985, 2.719934280785343, 1.9887944968444469, 1.2465067372508685, 0.49760685529298865, -0.2663750586123754, 1.472174330895207, 0.6840048245726109, -0.10416468174998528, -0.8923341880725815, -1.6805036943951848, -2.468673200717781, 3.026342600139216], [1.5338978306067297, 3.0615010404355054, -2.758393456663949, 0.8534647906498449, 1.0761506832613037, 2.6694518300714343, -1.6878506442007186, -0.4886765846812686, -0.2753272865886025, -0.5069606035193992, -0.7411365482174581, -1.325077022964937, -1.9105375512683125, -2.588669596294306, 2.9953313941921103, 2.3685666029962213, 1.6628570995208847, 0.947853727727388, 0.2607550341060403, -0.5317532404619847, -1.237018897609623, -1.9459679464344788, -2.6925456367267273, 2.8756016375309557, 1.9947456443606946, 1.2326692807511215, 0.5635306863327063, -0.26782948148636443, -0.9306911645137994, -1.6852666437800021, -2.488262005341241, -3.138671838387136, 2.300253834619303, 1.4862948550420487, 0.7985288509844759, 0.018541545827232664, -0.7385792666862852, -1.433332465365471, -2.152600292425079, -2.877995392802764, 2.577928298068702, 1.861548624754338, 1.1574253040103528, 2.7618894138756573, 1.9737199075530611, 1.185550401230465, 0.39738089490786876, -0.39078861141473453, -1.1789581177373307, -1.9671276240599198], [1.1416482312749956, -2.1224578653827315, -1.2419147205687757, 1.1196173726602936, 2.8438978422858625, -1.918658068653361, -0.26837050579078436, 0.9283703475242753, 1.1697553016203024, 0.9500153936936435, 0.6994416696690067, 0.09836305217661234, -0.533643412549111, -1.1404412343485895, -1.8294818282532788, -2.5318450538395183, 3.1244993373076646, 2.303742111589152, 1.6043845054095591, 0.8056843168974055, 0.1066795524176598, -0.5801977408359704, -1.3157012402503216, -2.0199768478093585, -2.9168859937068685, 2.6264502526814795, 1.9203284894260726, 1.1283815692775452, 0.44140905483793347, -0.36995109605795307, -1.0306052226979858, -1.7941988446642618, -2.557955073412912, 2.919703771290833, 2.210763673871689, 1.3919332210040531, 0.6756494537422673, -0.050032993554148586, -0.7843211815314666, -1.5407598989854376, -2.2827314774230976, -3.0466409502411373, 2.579170884110347, -2.2315808103234787, -3.019750316646075, 2.475265484210915, 1.687095977888319, 0.8989264715657157, 0.11075696524311951, -0.6774125410794696], [1.3706799712951998, -1.955872342516546, -0.3759571418964107, 0.9365644033956606, -1.7562522643551155, -0.2681470934981398, 1.227601616190917, 2.355513985660604, 2.5965820883129886, 2.446606350472287, 2.1329334477339117, 1.520500622508962, 0.8575124229721318, 0.30975539851479184, -0.3426410489897833, -1.1233588944173434, -1.7558129566238172, -2.621699245548747, 3.0323104742845075, 2.2553531445664525, 1.4992267718959091, 0.7877236125634361, 0.0740650673120058, -0.6446085826940227, -1.493493354392676, -2.221303553538533, -2.995331894340474, 2.5121294885707215, 1.7740044506552213, 1.0605455359157663, 0.38076247000627816, -0.4901111124979032, -1.1833660800228945, -1.9928258285794387, -2.6617629234639573, 2.767574846081339, 2.04072950313044, 1.3162093208226437, 0.6287512105351238, -0.1025200020000443, -0.8841586335942462, -1.6427964689097587, -2.3170690396072335, -0.9418657273430213, -1.7300352336656175, -2.5182047399882137, 2.9768110608687763, 2.188641554546173, 1.4004720482235768, 0.6123025419009878], [2.270052517717769, -0.6517859821048297, 1.2252421121186607, 1.1894120888430102, -0.5582282861522749, 1.3618033460552077, 2.6976906804842464, -2.466400010544408, -2.267366672305368, -2.3780717671675795, -2.765262137207287, 2.9062058725971696, 2.273777801890642, 1.6782887174253034, 1.0266991303446389, 0.21660021527163664, -0.3772155284532559, -1.1838680128817458, -1.8550055989786678, -2.601562506346564, 2.8617265981208284, 2.1606308971442623, 1.4803562491233357, 0.7449892946508676, -0.05166707008717353, -0.8429177311987424, -1.6070054329486396, -2.3839064741686045, -3.0401682408385398, 2.4846009529394664, 1.7152556262941818, 0.9322617911010731, 0.19840525131930598, -0.6181103310015956, -1.31398912491942, -2.1665191553363545, -2.8483768843636366, 2.6974371320535733, 2.026431065507193, 1.3325829771440905, 0.5859758309473424, -0.24972062021190844, -0.9631157919776387, 0.347849355637436, -0.44032015068516017, -1.2284896570077564, -2.0166591633303526, -2.804828669652956, 2.690187131204034, 1.902017624881445], [-2.74711425396789, 1.8597981374460595, 2.862433641893528, 2.825547981100126, 0.6164851347039182, 2.9648313045589525, -2.2294627812581815, -1.0526153134841714, -0.8204982757172026, -0.9515268099280014, -1.376898294697714, -1.9631720481996844, -2.5769172522432093, 3.041422831136206, 2.34366923941959, 1.6257339291449, 0.9675446811967738, 0.34470538593400946, -0.4259951340017949, -1.2369763995674745, -2.0121132843882883, -2.7602743392463047, 2.8911329889842143, 2.0632860302468323, 1.2084413158948166, 0.5594972457111282, -0.2209420128724684, -1.0098268286100485, -1.6524968827258117, -2.4037670517304477, -3.1227340512451196, 2.3101066701350312, 1.57718200649348, 0.7170073305894391, 0.060325848769466006, -0.7570635333853755, -1.4353075768895112, -2.199847049412333, -2.9006520612265314, 2.724462796814933, 1.96669934810188, 1.136142419410108, 0.42029055991111, 1.6375644386178934, 0.8493949322952972, 0.061225425972700975, -0.7269440803498952, -1.5151135866724985, -2.3032830929950947, -3.091452599317684], [-1.1398463702235482, -2.0432195715097627, -2.2715397661656844, -2.513050708006201, 2.454499826344584, -1.7469885352408987, -0.9158712640632878, 0.3944897621358443, 0.5833396607076899, 0.4187244064246691, 0.061417679464309316, -0.4884956985065294, -1.155663542809858, -1.7792788324856907, -2.47486408084664, 3.0250588558232785, 2.396411222790647, 1.8225531908012158, 0.9930765809135025, 0.20420123277848035, -0.6244230005640112, -1.3503535804664182, -2.017543674813446, -2.858791302085411, 2.5136386195539266, 1.8708054846528164, 1.2190244335387597, 0.3990600286684476, -0.268173547602391, -1.0581256934531886, -1.674512470861071, -2.586494237529788, 3.011163909465683, 2.100163369962445, 1.5151712645357804, 0.6904293000228332, -0.027007116407812504, -0.7743884556620486, -1.4908669711837543, -2.218624666177413, -2.943510563198263, 2.5246574255473684, 1.7795876800005708, 2.9272795215983436, 2.1391100152757474, 1.3509405089531512, 0.562771002630555, -0.22539850369204828, -1.0135680100146445, -1.8017375163372336], [-1.4568358346344148, 0.036663713903781314, -2.0816807817772336, -1.9387836154060487, -2.797949224129777, -0.2497407833594032, 0.5357610572220999, 1.8502731674519275, 2.0134328550167844, 1.8056105832412577, 1.5124184700556889, 0.9706648425986621, 0.25687931616290527, -0.37686819619129963, -1.0238386325164903, -1.8775938629626907, -2.533431763837129, 3.1098664637203584, 2.3257685253523626, 1.5870202416862256, 0.8280607258345647, 0.033968531852409, -0.6515687043057241, -1.501385002252995, -2.233709928049109, -2.9673475310764736, 2.5366895912837073, 1.8438261626294015, 1.2109915016258412, 0.33665212417687584, -0.3224347466726485, -1.1939326862355522, -1.8969733796136588, -2.7518682511520485, 2.9354114476881694, 2.0389812309498936, 1.3943311736042858, 0.5761292522701282, -0.14668552722922357, -0.7730853105004165, -1.4836511860292685, -2.3546422166649137, -3.140677616696509, -2.0661907026007924, -2.8543602089233886, 2.6406555919336014, 1.8524860856110053, 1.064316579288402, 0.27614707296580576, -0.5120224333567833], [1.0116622427306972, -1.6650696471746294, -0.09601465643471485, -0.4407791829561596, -1.957994750535402, 1.4102183537449484, 2.013367813752904, -3.0304536677269986, -2.778600786181439, -3.0052431132941386, 2.940213302095298, 2.3681514242552275, 1.6892748428195965, 0.9892892930037611, 0.3944268086549023, -0.5267558796814527, -1.1495785733033053, -1.8439632854372334, -2.619415468576136, 2.918930851300953, 2.223242696425565, 1.3973187834614507, 0.7179409234063172, -0.06548058491934938, -0.8778102545561026, -1.6013045024053874, -2.409797332722203, -3.0929392227783303, 2.527379715727065, 1.7504825034278433, 1.0292221602825258, 0.22843574286263646, -0.5648705578636157, -1.364495092312767, -1.9772015018267375, -2.7963747663770935, 2.759863474478241, 1.9604158968995478, 1.2361792832510332, 0.5213901060966837, -0.12785389742769837, -0.972304687861449, -1.7701083838563756, -0.7764756196203351, -1.5646451259429313, -2.3528146322655275, -3.1409841385881236, 2.3540316622688593, 1.565862155946263, 0.777692649623674], [-3.061442519713683, 0.16807784344308985, 1.3216664109834433, -2.146797136154003, -2.498533533426123, -3.0479961952555605, -2.718027804343418, -1.5917507924213474, -1.4234132742946422, -1.5935982585514772, -1.9159430533300217, -2.5431346022300794, 3.0402674808430312, 2.371141149216591, 1.6853266270299798, 0.9081840400536052, 0.23564292877373205, -0.426054406225866, -1.177067012669518, -1.901512274210038, -2.6491914913668317, 2.8324117594482274, 2.103288368734791, 1.250424709142397, 0.5285152935474642, -0.25314809417884376, -1.0559169119500353, -1.7922605310646489, -2.4645571851884824, 3.1245671671043738, 2.398885999360637, 1.5642421697296562, 0.8012400747920303, 0.019743259159620052, -0.6018410887491967, -1.4050388257539677, -2.163517165953868, -2.959095941264863, 2.54519023797833, 1.8866954748391471, 1.2089239773780918, 0.41920750352353053, -0.44761479217445377, 0.5132394633601223, -0.2749300429624739, -1.0630995492850701, -1.8512690556076663, -2.6394385619302696, 2.8555772389267204, 2.0674077326041314], [-1.112201982436762, 2.139555732965551, 2.6427354900771185, -0.2806824064240594, -0.796689825587034, -1.2708038118709588, -1.3021480094133402, -0.16538105420250915, -0.029331809914577178, -0.19736314248350695, -0.5974667772954341, -1.2212057010379134, -1.873944534660371, -2.5787645538440103, 3.0166149859050684, 2.353433411041113, 1.577855203998844, 0.960451488098645, 0.1518158281045352, -0.5973568467856332, -1.3859077623582792, -2.06296500460045, -2.8364942203029635, 2.58937949106004, 1.8914058020345657, 1.0549898692851656, 0.32545434261683326, -0.4992799196676643, -1.1199036092049255, -1.8342288418747614, -2.544441939086294, 2.9011584142447084, 2.118823245777474, 1.379325807659658, 0.6691297731215258, -0.09045004480006291, -0.8131364708742694, -1.6042213177682143, -2.360028653970506, -3.0327394343326795, 2.529766427969781, 1.7692870289572138, 0.9695682714064944, 1.8029545463405725, 1.0147850400179763, 0.22661553369538012, -0.5615539726272161, -1.3497234789498194, -2.1378929852724156, -2.9260624915950046], [1.0115698156010602, -2.200699320892671, 1.929212792923952, 0.8977538738328725, 1.6662819826346613, 0.5737366466884346, 0.06505449164606958, 1.1823617401646551, 1.234582694475879, 1.1565435561549187, 0.7171540821452034, 0.1559163329787303, -0.5495272163850622, -1.2142287880073503, -1.9209099478887204, -2.6359510299402444, 2.886242918366296, 2.2440694158629775, 1.3912249610924015, 0.6572712922282022, -0.04706892144836061, -0.7847335907977815, -1.5950487633906008, -2.3523035870131928, -3.1196827490515098, 2.3747213276283787, 1.6201676344619642, 0.8627189591714775, 0.1016124781420018, -0.5599195700496935, -1.295673571002581, -2.0801408543882154, -2.86787649329915, 2.6602762162808027, 1.9315844951569794, 1.2644523423275054, 0.4917847769653214, -0.3012850824775004, -1.0919575239991293, -1.826913549274705, -2.4647311362982087, 3.100960573174307, 2.312925518328699, 3.0926696293210227, 2.3045001229984265, 1.5163306166758304, 0.7281611103532342, -0.06000839596936913, -0.8481779022919653, -1.6363474086145544], [-2.891182971026648, -0.480789924214168, -2.7688012390886065, 3.1237513447398904, -2.9701358666313276, 2.200173118183276, 1.4388165125528651, 2.5424626569011686, 2.6117727523940353, 2.3864403843253434, 1.9614914488420432, 1.3852809871816696, 0.6876666622598826, 0.0763697220618802, -0.6762646572785265, -1.4937388259645878, -2.1873482489997436, -2.8381332174731995, 2.6352681956268214, 1.9040894110786226, 1.1560394176346698, 0.36840411309087173, -0.38443978641393883, -1.1178340261963413, -1.9446175268857218, -2.721863616922917, 2.7822929275229242, 2.1269706580761145, 1.3294140688125644, 0.6403340159835977, -0.10368766797440543, -0.8621531301433301, -1.8572206366934516, -2.4157912295721893, 3.1311305378048218, 2.4516492189339196, 1.698708032559363, 0.9272773012189717, 0.10979867235725571, -0.5230439077252207, -1.3477255620257935, -2.0262084590082843, -2.729243427520027, -1.9008005948781062, -2.6889701012007023, 2.8060456996562877, 2.0178761933336915, 1.2297066870110882, 0.441537180688492, -0.34663232563409707], [-0.3741068283283546, 1.4285992278334838, -1.5246139989125744, -1.5485176020169469, -1.4063439665421988, -2.445881873111478, 2.7155887750232814, -2.5261058967438608, -2.4888270080415857, -2.7997312833172323, 3.127891530331812, 2.4326018246317496, 1.7944683155615344, 1.1046974183386276, 0.4645028968655929, -0.34973920249686685, -1.1098810477944347, -1.783830230142133, -2.541223946984804, 2.987474523820474, 2.3002075320422506, 1.4751078899029757, 0.7678754003808699, -0.013266335976595656, -0.8453689868755738, -1.578615465191266, -2.2878799305256656, -3.0843112844413447, 2.453002706878408, 1.752769986082047, 1.0225658967172357, 0.2062147441840665, -0.6422851643254788, -1.3317024390678327, -2.0671698319814595, -2.7641057826479773, 2.8381245169598266, 2.0703531368635097, 1.236280783487448, 0.6128530077127827, -0.21543669584339753, -0.8878951534012351, -1.590634087300712, -0.6110855118976488, -1.399255018220245, -2.187424524542841, -2.9755940308654374, 2.5194217699915455, 1.7312522636689494, 0.9430827573463603], [1.312545567911581, -2.9156894347297246, 0.14733025755536389, 0.031852655989776935, 0.40228503822354966, -0.916966497614812, -2.482386718655153, -1.4885332979601493, -1.4591838055842494, -1.7711600503176221, -2.229881718113294, -2.911817311986585, 2.685637690925663, 1.9582508127209373, 1.408781220624892, 0.5926583294787982, -0.19085382654786187, -0.8889438226390176, -1.6130188744336884, -2.363609128397602, -3.085374822654618, 2.3832837648696916, 1.7065312331446663, 0.9217834580832509, 0.11271072318783482, -0.7239376238064956, -1.3670142173206727, -2.2157634412954508, -2.9270185973488445, 2.6630619064487036, 1.9367030588744498, 1.0894007815644748, 0.36667110337745257, -0.4255907626439779, -1.090998270337714, -1.8053208377224124, -2.511223560609807, 3.0014829435350343, 2.2179206035830603, 1.5641430339752098, 0.6919701879998961, 0.07110366004810231, -0.6922869330981296, 0.6786295710828085, -0.10953993523978767, -0.8977094415623839, -1.68587894788498, -2.4740484542075833, 3.0209673466494067, 2.2327978403268176], [2.7273155491185115, -1.2923780879404738, 0.3266810855632336, 1.1534518281398896, 2.1477633135474257, 0.41672353700895925, -1.7498699078961018, -0.8419289755463844, -0.8381691503318542, -1.1121261593715879, -1.6203985170975024, -2.446159409544368, -2.970306206646601, 2.51753459079632, 1.9685767568747856, 1.1148201692809643, 0.407935449799286, -0.3430673557033366, -1.1167779528538766, -1.7675394305391698, -2.412268097288102, 2.9974308104407577, 2.2650571019084786, 1.505397104548674, 0.742689809997426, -0.023804330377007688, -0.8458174865474071, -1.5803983955133312, -2.282296330449139, -3.0141162981798537, 2.632335935563926, 1.7503633375454157, 1.00912280421322, 0.17717514334803397, -0.47912485911000147, -1.1300095479306584, -1.8891445975559762, -2.6474970736238816, 2.8761269526054, 2.2388378954205983, 1.4552154754018254, 0.8084045772027935, -0.035458610041771976, 1.9683446540632588, 1.1801751477406626, 0.3920056414180664, -0.3961638649045298, -1.1843333712271331, -1.9725028775497293, -2.7606723838723184], [-2.151243105215766, 0.1347908845441914, 1.9420787371668347, 2.9040655977684047, 2.7524039106931717, 1.1239769742875687, -1.6035465291965103, -0.667407965460999, -0.7548224143611613, -1.0551960131978753, -1.6767824566418632, -2.921977385774017, -3.053908662546494, 2.5685373561644305, 1.9220017766872566, 1.125399482792293, 0.45777707387890487, -0.3347994370116929, -1.394060762086692, -1.7802818604372952, -2.4652933178033827, 2.9708848582363423, 2.321520302238408, 1.572027206870768, 0.8011837014486325, 0.031004290805821455, -0.6865162341366933, -1.4281604432091832, -2.1768920426017395, -2.8615056258016978, 2.7221076434950753, 1.9411565964041735, 1.1879555340375383, 0.3830415935884055, -0.3008471538830726, -1.0282641151058023, -1.7627622971114754, -2.442315417315058, 3.061619128217341, 2.4396520401231214, 1.7326784890996656, 1.0770924729744493, -2.236956063813281, -3.0251255701358772, 2.469890230721113, 1.6817207243985166, 0.8935512180759204, 0.10538171175331712, -0.6827877945692791, -1.4709573008918682], [-0.1794882849893007, 1.7579657198217866, 2.8347041520341456, -1.4372393435311146, 2.670528038249639, 0.8716229217259404, -2.331702617557365, -1.3233871523388707, -1.4387886563826875, -1.7278527960987624, -2.404725488899974, -3.0819606234217396, 2.3937445109218665, 1.9136487827200916, 1.163732490263289, 0.4444280376998968, -0.26780150798975555, -0.9975371671723927, -1.746436706457711, -2.398626329310243, 3.087393707374769, 2.3427288300863545, 1.6600184045184925, 0.8906192487060416, 0.09804081469046011, -0.662972373254366, -1.3303046649733794, -2.1078929264906314, -2.828032407966063, 2.806862040707724, 2.0995273702018196, 1.2642258047770802, 0.5346691938466499, -0.26071351923685526, -0.9466666261464027, -1.6559250113429194, -2.3779632401436253, -3.0976978018374552, 2.5374140969862857, 1.882141491984445, 1.1822347165405382, 0.4758955106037206, -0.9472409808328237, -1.73541048715542, -2.523579993478016, 2.971435807378974, 2.1832663010563778, 1.3950967947337745, 0.6069272884111783, -0.18124221791141082], [0.7871868292899116, 3.030546510899473, -1.5827259362029018, -0.978519470009001, 2.648093633730465, -2.1892954210588975, 1.4779379047320695, 2.512727078261374, 2.41065015753372, 1.9338574202409369, 1.2517628319036156, 0.6716988172265097, -0.24975757974955926, -0.6820496933571896, -1.5049571579358805, -2.1250474197435985, -2.7991319942129316, 2.781951827130076, 2.138879927387226, 1.4832483067207285, 0.7864822812698584, 0.006872807367063416, -0.6034409632771762, -1.3287944721684788, -2.0445511917911965, -2.755844962889963, 2.8317310230125905, 2.128988326168521, 1.5079448484116078, 0.7974960449115649, 0.21228634505835586, -0.6161241688808055, -1.3820566021413718, -2.0822512095544745, -2.6231416619060646, 2.88550591920135, 2.214025909592749, 1.417186090566986, 0.8937870416198379, 0.27898830633071015, -0.43587506226303674, -1.1078617947490237, 0.34247410214763363, -0.44569540417496256, -1.2338649104975588, -2.022034416820155, -2.810203923142751, 2.684811877714232, 1.8966423713916356, 1.1084728650690465], [0.24404954803162937, 0.4983307270037365, -0.0016500855629537625, -0.7387972542457497, -1.2641565489448077, 2.9648835050641473, 2.5454228341018954, 1.9279930684580044, 2.2267959048758392, 1.454705591148521, 1.4639728087911656, 1.0473163695744283, -0.47228853053842457, -1.324563158123997, -0.6936894897820629, -1.1169694839687203, -1.713441337785273, -1.862685002730661, 0.04637125000958875, 0.7500609466147274, 0.6021683582685746, 0.41112896757914896, -2.159984668482931, -3.0834085201215053, 2.541378288302848, 2.088817407112824, 1.405738465126884, 0.5188945503491347, 0.9242795491786033, 1.022585445815988, -0.7277778570794204, -1.9958472852769127, -1.5667698721270291, -3.089620401287089, 2.2166451043866147, 1.5831382620268357, 1.025850023448136, 0.6716339373738656, 0.019655220937309537, 0.08544333114841862, -2.9846767369663034, -1.430313902334163, 1.6321891851280839, 0.8440196788054877, 0.05585017248289148, -0.7323193338397047, -1.520488840162301, -2.308658346484904, -3.0968278528075004, 2.3981879480494968], [-2.278297316809631, 1.388490346931352, 2.6542166374114267, 0.15397289456136676, -0.7904226585563343, -0.5883490356793963, -2.404375275446622, 2.5798395730558745, 2.493418939552992, -2.988509322952165, 2.982208596826549, 2.2864372640120756, 1.0419538679814444, 0.7238165753473247, 0.7337070284111995, 0.38690709828894043, 0.0927838661589071, -0.09203916763607722, -0.8188616600687375, 1.3254634141425363, 0.8524994695910983, 0.3841501806699519, 3.011119646688652, 1.1663030342060843, -1.91905020417067, -2.8105260252833055, -1.1132177089986008, -1.371204312612388, 0.36836227098430285, 0.6199274004920134, 0.014203956559487807, -1.7668193187534236, -2.0092617581403367, -2.650987458546684, 2.652159436977616, 2.370292565439396, 1.4371554023777975, 1.0498416034891669, -2.3489031060890007, -2.4408347367728744, -2.918012149006966, -2.7089810949945914, 2.921904268108541, 2.133734761785945, 1.3455652554633488, 0.5573957491407526, -0.23077375718184356, -1.0189432635044469, -1.807112769827043, -2.595282276149632], [0.18530838161209928, -1.676619293836243, -2.8300694149538863, 2.6546443759726976, 1.7800712606230213, 1.3901345051742204, -1.5206266893800766, -2.598250398787396, -1.669340703161165, -1.6783821515324568, -1.8531426417728873, -2.5837344931407777, 2.2391843645459595, 2.0474385051039796, 2.1792865620186284, 2.0520492066823657, 1.7903633263847176, 1.8144485650332136, 2.4585454352466947, 2.5714164750711355, 1.3836935680175522, 1.1236309718927409, -2.291853960933995, -0.5648777719091775, -1.0342255774076925, -1.3907006232151353, -2.959913171983583, 2.2691431171918843, 2.355255063259161, 2.1834467042416428, 1.4113370373563576, 0.5210321178926556, 0.30687048946498763, -0.6403429712011182, -1.6703713559269424, -2.4754248689834277, 2.437397375403094, -0.3955860513535079, -0.5351262786296473, 2.8163633438135953, -0.40135244920017143, -1.939256445270182, -2.071565956090595, -2.859735462413191, 2.635280338443799, 1.8471108321212029, 1.0589413257986067, 0.2707718194760034, -0.5173976868465928, -1.305567193169182]]
  in  "SerialNumber Z":string="26004283"
  in  "KCubeStepperControl Z":refnum<k24>(container)
  in  "Num Of Steps X":i32=50
  in  "Num Of Steps Y":i32=50
  out "Amplitude":dbl[][](graph)=[[0.009909326858225397, 0.007447072438705031, 0.006863630798634195, 0.0014695705947812107, 0.002220842274561089, 0.01626715578847811, 0.17085384478189736, 0.23548832292415753, 0.27800774958716157, 0.3136647096076685, 0.33493465977172393, 0.33789368695180405, 0.3373544170380455, 0.3475362604565154, 0.34874739872171173, 0.35133323434446107, 0.3538846890806939, 0.34512932141592206, 0.32867248501470114, 0.3499583480314827, 0.34898084299092047, 0.3489190696286534, 0.3464812384824027, 0.3472066497060785, 0.33662226610943874, 0.34184428230950886, 0.3444876339687898, 0.34252363850815654, 0.3404185061565854, 0.3360663801785765, 0.34318921524815726, 0.3373364482521718, 0.33778396549974454, 0.34631313473653547, 0.33356299677038526, 0.3348730552587252, 0.32775895781179193, 0.33397425175134643, 0.3263941718565294, 0.3383965102136854, 0.32836482268073564, 0.33323430904122353, 0.32732332624260174, 0.0, 0.0, 0.0, 0.0, 0.0, 0.0, 0.0], [0.00712099769046828, 0.009978587968371385, 0.005091610443354114, 0.0075322059839166644, 0.0029312465944280114, 0.020636302344694643, 0.19265289810357986, 0.24462236684837377, 0.28698327968315096, 0.3115113642757042, 0.353401284251413, 0.3477686103779527, 0.3507317160062189, 0.35617294657011694, 0.36024397921801815, 0.3589769574996201, 0.36377268890363523, 0.35413622574541065, 0.3586356658209888, 0.3533368134200202, 0.36363849137250276, 0.3601086373609252, 0.35192200012141, 0.36102645030191, 0.22427721808294818, 0.2913841482409055, 0.3553129130781941, 0.3514285969148294, 0.3520507696572119, 0.34806202201650355, 0.35023782889325866, 0.34982445255741257, 0.34937941179388365, 0.35193301706684255, 0.34503703467773233, 0.3459803596864817, 0.3416657184518222, 0.34379904173264764, 0.33958551730432596, 0.3467584798350045, 0.3420672808718163, 0.33986564015711024, 0.33890650620513235, 0.0, 0.0, 0.0, 0.0, 0.0, 0.0, 0.0], [0.006727875108310154, 0.00922791256742799, 0.005419655623166341, 0.006305387021503958, 0.005558462572538865, 0.02042120165239349, 0.19236079431687433, 0.24462120561219364, 0.2893326872330407, 0.3164415216961298, 0.34850001304094785, 0.34562572223257837, 0.3575195353240587, 0.3626763396913711, 0.3582544399713563, 0.3573263853368624, 0.363598348500192, 0.3542862999643566, 0.3578383666922749, 0.3603630233196922, 0.36465728516185053, 0.3567159512284138, 0.3562574396920364, 0.36053743608948324, 0.273495317207077, 0.3194783574659899, 0.3578859976625434, 0.35450014258071244, 0.3467879870325758, 0.3482821226723854, 0.34936394862068904, 0.3479865043839947, 0.3498887914333911, 0.35208570512911586, 0.3455516693288507, 0.3469072841035606, 0.34232043575669996, 0.3412912965699265, 0.3393634038892212, 0.34409253899928754, 0.34363780112516207, 0.3410575938636074, 0.33959008118593764, 0.0, 0.0, 0.0, 0.0, 0.0, 0.0, 0.0], [0.011526074711152478, 0.01452314655808943, 0.010288385234886717, 0.00460166423029998, 0.005749939527699393, 0.019299764837971453, 0.19830939712401732, 0.24332164241087034, 0.2969506435247628, 0.324094995497271, 0.3464328230563815, 0.34699509583590826, 0.362875140827449, 0.3630664941840688, 0.36351689669930837, 0.36906484133485473, 0.36660584384029093, 0.3622154282694259, 0.3530284622933743, 0.3644987085874467, 0.36369287848513526, 0.3622996096880689, 0.3622110159667562, 0.366738212033477, 0.3627269424161541, 0.3612887395232012, 0.35998593981681154, 0.3546784005999543, 0.3533534633031919, 0.352211066456362, 0.34856048138900614, 0.3531492779774996, 0.3513090270549004, 0.35016495949960025, 0.34384237886454394, 0.34694120307737986, 0.34267127522484114, 0.3408261179079747, 0.3431509368849641, 0.3446098520419354, 0.3452402015176513, 0.3431393227640425, 0.34436272838231563, 0.0, 0.0, 0.0, 0.0, 0.0, 0.0, 0.0], [0.016600652113197112, 0.008573418820702483, 0.010023659901021517, 0.004229935833059878, 0.00231407678580869, 0.015933606952155954, 0.1995328012119833, 0.24863925704249143, 0.30276181914039857, 0.32764719683245147, 0.34509291358148314, 0.35041971677984374, 0.3625281077351741, 0.35653703625688987, 0.3584701962313671, 0.36919784910276476, 0.3660518725952989, 0.36047074719715544, 0.3388964690179368, 0.36288115201378285, 0.3599461642976939, 0.3607290680545271, 0.35880678813632777, 0.3617930467653677, 0.3681162010870813, 0.36443453222842137, 0.3622152918071352, 0.3597122707699377, 0.3517063610000002, 0.3521023922855256, 0.35278321200374857, 0.3534026732664232, 0.3572965066262747, 0.35192922823187717, 0.3490519893327172, 0.3464205955057271, 0.3457500973132356, 0.3430484815278443, 0.3478564163753748, 0.34895626501248445, 0.3454434544249081, 0.3466476777539285, 0.3429953538308366, 0.0, 0.0, 0.0, 0.0, 0.0, 0.0, 0.0], [0.017334228732931396, 0.006874329438346918, 0.009869481079350375, 0.000992757066557687, 0.0025918839264460277, 0.019371388766765626, 0.2075878296394193, 0.24976734116392962, 0.30701183419259986, 0.3278423770258674, 0.35298723048746666, 0.35016396169116315, 0.3641844081643669, 0.3682040104148031, 0.36566096336362347, 0.3670654089456184, 0.36891213722247695, 0.35967879012476783, 0.24853793143489694, 0.36595032320464166, 0.3617048488068905, 0.3630713999609799, 0.36224722123978764, 0.360814961394152, 0.3670882308390812, 0.3650157735832273, 0.35949931701452925, 0.36328561889871963, 0.35242558294729337, 0.35254924393661524, 0.3495438308921983, 0.31011589885954216, 0.35735297031417623, 0.3551136176347853, 0.35031017219600463, 0.3474387820402967, 0.34728359428380756, 0.34507811058940024, 0.3479505016399615, 0.3448320863371714, 0.34636105641710924, 0.34531340186966153, 0.33782367992279966, 0.0, 0.0, 0.0, 0.0, 0.0, 0.0, 0.0], [0.016398879961867976, 0.006397499396715778, 0.009065122304491241, 0.001186578952188264, 0.00367391703013349, 0.03552994823945723, 0.2114231035999929, 0.24970335757988443, 0.3074705035340807, 0.33245127715664774, 0.3535753174123768, 0.35188988045640124, 0.36443685339886805, 0.37184462666432694, 0.3613552855057262, 0.3690035499118032, 0.36759664385341523, 0.3582064365570069, 0.3169831585107266, 0.36720148472894837, 0.3613038682187626, 0.3638547712641863, 0.36134346745895723, 0.3611124276164479, 0.3659488688321944, 0.3640157120624338, 0.36859134493318735, 0.3630258149453095, 0.35181107251646443, 0.3528875571607901, 0.3485290962953736, 0.3276563959239802, 0.3589113938436776, 0.35254918932663276, 0.35102675321761695, 0.3494729783209572, 0.34494680843283515, 0.34699294761777283, 0.348157778391929, 0.3430908350314865, 0.35016004058224537, 0.3417519537798013, 0.3398681981862596, 0.0, 0.0, 0.0, 0.0, 0.0, 0.0, 0.0], [0.013172336665812754, 0.009195185878744608, 0.01787782559798046, 0.017556327668343547, 0.0303769829129266, 0.052722392431721374, 0.22230354125762486, 0.24867132335508707, 0.30438759366027063, 0.33427976972868034, 0.3555507996085605, 0.354336235282706, 0.36725678283867946, 0.3683135127103853, 0.36530232113914346, 0.3728928980809481, 0.37119551625653474, 0.3663253554694902, 0.363503507199729, 0.36237955846884423, 0.35841463705701154, 0.37229572434355784, 0.3611291825035545, 0.3635670973264331, 0.3711767732063333, 0.36388839064501766, 0.36556976220875975, 0.3590805764310172, 0.3543355029967816, 0.35371321427729174, 0.3581366789412586, 0.3561546016208726, 0.3555725063492627, 0.34954258309602076, 0.3515083336768137, 0.35133267798341694, 0.34215627649007474, 0.3498278863807251, 0.34707907082442013, 0.344412780005518, 0.34652726806425654, 0.34496177587666166, 0.3409581541115369, 0.0, 0.0, 0.0, 0.0, 0.0, 0.0, 0.0], [0.013157238237033492, 0.006865929637368289, 0.010290428352944168, 0.006453777738371383, 0.006559489561382754, 0.04146228237115531, 0.23334696604979513, 0.25003046406559915, 0.3056827539408604, 0.33447797660356865, 0.35312332755494086, 0.35806364405509733, 0.367105123984707, 0.3712628388398568, 0.36538871429419967, 0.37136718345258984, 0.37125287442183397, 0.36546294913020977, 0.3646207762104281, 0.3546402202719004, 0.2642217076433554, 0.3637438620081864, 0.3574649562930537, 0.360299339990991, 0.3746742466434918, 0.3629418955900367, 0.3633924509769665, 0.36141082268476277, 0.35214826905804725, 0.3550118397447968, 0.35388318669535607, 0.3585002606102065, 0.3522715355442067, 0.35419784917698527, 0.35139473131528914, 0.3497807535605884, 0.34342616954161703, 0.34805105530860847, 0.34393842728405055, 0.34323289927575795, 0.34256026461786504, 0.3434293540939328, 0.3396613237880671, 0.0, 0.0, 0.0, 0.0, 0.0, 0.0, 0.0], [0.005303454614768298, 0.007877033454687593, 0.008694157711653534, 0.008383296429753504, 0.014247635266676214, 0.03997505325508367, 0.23666353618462987, 0.24995333447117377, 0.31265673808676037, 0.3368370195500952, 0.3549886395783624, 0.35983721265830987, 0.36831122010744954, 0.3710892347761823, 0.3680581879918959, 0.3693185353145501, 0.3680704159684521, 0.36570993986697314, 0.3658900448830211, 0.34258702150640663, 0.19927540861652823, 0.33563686903112516, 0.3637011646513705, 0.3622564581648499, 0.3709144046030079, 0.3646950258288415, 0.36407612498126873, 0.3596059273523912, 0.3501985065060999, 0.357048694418594, 0.3561366628920939, 0.35714972424436287, 0.3545703977082046, 0.35569316932858575, 0.35024154613485414, 0.35162761620345345, 0.3446929451494764, 0.3440337039125173, 0.3430991245163142, 0.3456137493467753, 0.3431064242284195, 0.34522587912983543, 0.33734448758694674, 0.0, 0.0, 0.0, 0.0, 0.0, 0.0, 0.0], [0.015272208295267539, 0.0063713442743622214, 0.010351855421121806, 0.006453052406911673, 0.014729482244262914, 0.032872451494759765, 0.2445921833731899, 0.25495042942512125, 0.31302913543456923, 0.33706868101564785, 0.36061838544746055, 0.36043092459763193, 0.36887453485328914, 0.36968674475759855, 0.3690902878039094, 0.36672970552580125, 0.3697227798748303, 0.36366154535262357, 0.36531016802832966, 0.3629630298467638, 0.35317173126004003, 0.3428411251509001, 0.3584597797103456, 0.3603527791561164, 0.3679396477917944, 0.3645775231283353, 0.37055194996405627, 0.36501796306243334, 0.3509015796681946, 0.3541440487896163, 0.3601203572592975, 0.35607168141677564, 0.3543298201385417, 0.3559446150792338, 0.3537906539042604, 0.3501059372162014, 0.3489190612689992, 0.3482858367582495, 0.3494712666593778, 0.35014613969211067, 0.3476240126595215, 0.34878292706403324, 0.3391804212955978, 0.0, 0.0, 0.0, 0.0, 0.0, 0.0, 0.0], [0.009595291902339176, 0.0038674809115718453, 0.00940598861126335, 0.002758530739748405, 0.010323318681070974, 0.033719331416005534, 0.24452209291511984, 0.263708519668499, 0.32023068876707633, 0.34247709542712623, 0.35961399070819217, 0.36199048501801706, 0.36887100165740305, 0.3723420777454854, 0.3672366199506962, 0.3671259896788317, 0.3711558540230388, 0.3661689111496352, 0.3635866844024856, 0.3673173728309849, 0.36009800269902414, 0.36929547601170265, 0.3615995960900538, 0.362275306569596, 0.36611740742884946, 0.36494301866641415, 0.3648530489630222, 0.36536587359166683, 0.3566482653338253, 0.3555595012419955, 0.3543029232933589, 0.3524079794703638, 0.31360745679631424, 0.3642494563064474, 0.3521837149134609, 0.3512418621282264, 0.34931514936003105, 0.35023424827665334, 0.3537924479488913, 0.3445534354485487, 0.3517484228686984, 0.3464305833017441, 0.34644521849793236, 0.0, 0.0, 0.0, 0.0, 0.0, 0.0, 0.0], [0.015081075295961649, 0.006478856791829531, 0.0069903768811867975, 0.0015994315112272377, 0.00821423935740475, 0.045552402530362066, 0.2526372285611156, 0.27165518382862197, 0.3289137070292543, 0.34539524981074043, 0.3597257225590577, 0.3615341927868585, 0.36465918110599116, 0.36946223899282177, 0.366530259191182, 0.36716489218849296, 0.3722317713463965, 0.36649797001381346, 0.3663061999099886, 0.36782123478958906, 0.36598955672719263, 0.3694214840260906, 0.3619728412899513, 0.3555819775887321, 0.3694321567746621, 0.36626276990940665, 0.3699879884300565, 0.36577772983480666, 0.3565659027541401, 0.35764728716767624, 0.3612777470615022, 0.360472507996689, 0.39085838232100617, 0.3242842004600711, 0.3531676883202306, 0.3523991279855241, 0.3475464623008839, 0.3484509828744777, 0.35373706342402755, 0.3451396058197649, 0.35291664433649556, 0.3460249790878955, 0.34320590573672954, 0.0, 0.0, 0.0, 0.0, 0.0, 0.0, 0.0], [0.00854651787932253, 0.013493238115178219, 0.002700595811491519, 0.006549600615902305, 0.0044843412091418585, 0.044865736264070706, 0.25749136053107885, 0.2718576416824315, 0.3367576104571059, 0.3531202780001589, 0.36457815706576685, 0.3639404629994585, 0.3658200182416614, 0.37443122443125376, 0.36830900747523765, 0.3694938870410978, 0.36919635991069377, 0.37003217194874627, 0.36794136570930047, 0.3666531126521246, 0.3606333472590198, 0.3656471934288562, 0.36594128947650195, 0.3648441045330962, 0.3715075306174503, 0.369341612088188, 0.36971818578559523, 0.3634766366441, 0.35670299649183884, 0.35758534158111166, 0.3602452361279215, 0.3620915314160378, 0.36053613075577734, 0.3618119995637294, 0.3627301613098807, 0.3514931000628217, 0.3507128039985892, 0.3501262668866027, 0.35728093088606483, 0.34546513529579603, 0.35733184569210585, 0.3463312817839891, 0.34539063774362533, 0.0, 0.0, 0.0, 0.0, 0.0, 0.0, 0.0], [0.01013900003090122, 0.0034533554708371383, 0.007327816640900558, 0.004649803304028705, 0.004353966141802266, 0.0557114600119526, 0.2513447400339754, 0.27780489637686595, 0.35028676825465055, 0.3602862693916891, 0.36636294467530867, 0.36294459641284066, 0.3654472494473204, 0.37247178483655025, 0.36593156311305713, 0.3671074290987575, 0.3718514250619294, 0.3753298549092542, 0.3590801165357297, 0.37179141463537557, 0.3704218565451305, 0.3674324192024468, 0.36505910947275605, 0.3624631959158577, 0.36640691079849536, 0.36793415013731884, 0.36684799575232274, 0.36397013674984124, 0.3592862816092317, 0.35575993355546837, 0.36444674811367006, 0.36369407001973797, 0.3647627316979603, 0.359487926489682, 0.3577805751032349, 0.3548704711645606, 0.35527060128611426, 0.35450458626925835, 0.3541204510326463, 0.3500076709985456, 0.3562388343852543, 0.3520451845770609, 0.3473378962302747, 0.0, 0.0, 0.0, 0.0, 0.0, 0.0, 0.0], [0.008161558536840845, 0.0038798902132368054, 0.00589256103770034, 0.01030973325474141, 0.004839216927926541, 0.044008702345279954, 0.2201320210274993, 0.27030115668757976, 0.3524549404218326, 0.3649610324172724, 0.3680164766655046, 0.3636955353121344, 0.36453103486419713, 0.3723246223013763, 0.36536850755182054, 0.3675564092651077, 0.37237299338873175, 0.37022074183879766, 0.36200043046462055, 0.3634966569616632, 0.3696216415075482, 0.36816622648156855, 0.3655013072294447, 0.36452049838452844, 0.3655460727603323, 0.3698893014090151, 0.3723605591120664, 0.36669692191474307, 0.3590626240939363, 0.3604896476716108, 0.36435684263173135, 0.36814141677066825, 0.36385945006556625, 0.3573622197526283, 0.3583031068469389, 0.356438010702074, 0.3570240717373364, 0.3566348906287026, 0.35852056163602586, 0.35174932877082454, 0.3524474571000907, 0.3565511933091859, 0.34752668443212253, 0.0, 0.0, 0.0, 0.0, 0.0, 0.0, 0.0], [0.008641630846475713, 0.0038251143930674684, 0.0014715891139254237, 0.0038758452792154578, 0.014335727782436124, 0.04669294421144401, 0.22402469718280812, 0.2487046624777815, 0.3317977906317034, 0.37214035616291574, 0.36563577496963495, 0.36397584652946785, 0.3677147705145585, 0.3698791430931084, 0.3660356356544713, 0.36543427574545345, 0.36987844413078885, 0.36690351390955056, 0.36299590021276024, 0.37164086464750334, 0.3687473150746952, 0.37155153317081174, 0.36291653505329946, 0.3658964918031467, 0.3692379415430509, 0.36802445314622767, 0.37252303600974, 0.3715294946726244, 0.3587690676675567, 0.36028370533060633, 0.35633028903500946, 0.3701585978649001, 0.36271750281255943, 0.3604759131365399, 0.36247073420815384, 0.3567776440577493, 0.36021939297331573, 0.36293736179856484, 0.3619867629454668, 0.3588680455831806, 0.3541951386864591, 0.356665232250383, 0.3514462719856032, 0.0, 0.0, 0.0, 0.0, 0.0, 0.0, 0.0], [0.0093009554008974, 0.004286611207806374, 0.002847726739404292, 0.002490520630324693, 0.0100217633266386, 0.05421817708984437, 0.23380056425152304, 0.25043539153030125, 0.3199141897848126, 0.3619868576093946, 0.373875947041048, 0.359861336522623, 0.36865117881586223, 0.3712443915755383, 0.366781429717893, 0.36759311725019744, 0.3736685420924964, 0.36721515655594966, 0.366080984681913, 0.37141493451928814, 0.3710485738508909, 0.3675770968283141, 0.3675795354805305, 0.37311790763799546, 0.3698585822073598, 0.3658766107241295, 0.37350223816894607, 0.36584019776970605, 0.3654672311972598, 0.3659082116814189, 0.36546995154630135, 0.3684632088664309, 0.364957225204692, 0.35982865717242096, 0.36521715286391027, 0.3604687735699779, 0.3605172701334213, 0.36464297348856417, 0.36078092431759146, 0.35656094502571534, 0.35907894687687414, 0.3536751733774806, 0.35227536715463087, 0.0, 0.0, 0.0, 0.0, 0.0, 0.0, 0.0], [0.007288634560850498, 0.004474448484652666, 0.0046968418194584995, 0.0023811585558207986, 0.003188943957836061, 0.06244219421680429, 0.242269965197806, 0.2507575785593998, 0.32232257547387927, 0.3492133237148299, 0.37258583727324796, 0.36318052081985464, 0.36852789521686297, 0.3715411529341363, 0.36805421294752233, 0.3693014765132082, 0.3758321628760945, 0.3692498849110293, 0.3666709461928248, 0.371322137686725, 0.365789809066605, 0.36865939025808325, 0.3700832635224179, 0.36774315578333844, 0.36571066282927656, 0.3668793444210761, 0.37205267220102906, 0.3746002149472588, 0.366874358574067, 0.3680874453702782, 0.36286728105019334, 0.3702643335687224, 0.36892531100789927, 0.3109312494293619, 0.36778007037837784, 0.3576386147993654, 0.36197380443176197, 0.3607220165816636, 0.36348110669105765, 0.35822005025664205, 0.35992563856089066, 0.35512032641333957, 0.36145476861660125, 0.0, 0.0, 0.0, 0.0, 0.0, 0.0, 0.0], [0.0070373725857065415, 0.003578491460065517, 0.00696118504865266, 0.003625530638913065, 0.005557575073108958, 0.06832951868711593, 0.22184160923381677, 0.2707114690994966, 0.326014927700834, 0.35347463462601786, 0.3609833745517803, 0.3683618987868989, 0.37192514639602053, 0.369334202915946, 0.3693171378441848, 0.36458822382246453, 0.3725513257373612, 0.37272085264197247, 0.3660390644180457, 0.3715870547013901, 0.3618207673380088, 0.37303392135068375, 0.37488129410296966, 0.36947515928667535, 0.37054335260453125, 0.37496620669004105, 0.37080684399369174, 0.37449168832200536, 0.369344112202341, 0.366819597732564, 0.3652184276598851, 0.3717910732685973, 0.36847304179143336, 0.3761726598212409, 0.30470639863853105, 0.35801641155920066, 0.3631851902372165, 0.3633016433476309, 0.3669403746221117, 0.3625783760040312, 0.35936230317276313, 0.35888285174999773, 0.3618779810142058, 0.0, 0.0, 0.0, 0.0, 0.0, 0.0, 0.0], [0.011093725015822604, 0.005838724221745851, 0.0025902499586619083, 0.005766264224307911, 0.00785426221262095, 0.06359742535003085, 0.20470709993977987, 0.27546870997287726, 0.33478981878304226, 0.3512251258706148, 0.3604612947843715, 0.3612227623094815, 0.37144038705226395, 0.3735592298620856, 0.36508241094779265, 0.3714973469548542, 0.3663584012357174, 0.37278671364824095, 0.36334182442269025, 0.37117561304413615, 0.37492299281525965, 0.373377021573734, 0.37277581137744864, 0.3680590797265647, 0.36733424428862843, 0.377055977761101, 0.3762103119448772, 0.37352189228510096, 0.37055282428840136, 0.36998900201381796, 0.3669372008698421, 0.37808167032779894, 0.3716533611469102, 0.37356598084165454, 0.37395059461418434, 0.3632207903430957, 0.3656464710913062, 0.36603560315610684, 0.3651767639379295, 0.3616821732015765, 0.3625351993108309, 0.366305561258395, 0.3600596763088303, 0.0, 0.0, 0.0, 0.0, 0.0, 0.0, 0.0], [0.007759339616844029, 0.014218873209420441, 0.0017523427258162643, 0.005160267903319662, 0.007003756745731073, 0.0674180556406698, 0.1979264368164561, 0.2596672736983023, 0.34755716124246133, 0.35632311873587, 0.35670951049705785, 0.3591567952255285, 0.3705294056811745, 0.37536323430848345, 0.3722986155025629, 0.36736615050653915, 0.3717719265308364, 0.37675288190089534, 0.3647504114942438, 0.36843669205080404, 0.3763629820310433, 0.3734259602498128, 0.3751613114306013, 0.3746961846137674, 0.3694996222414408, 0.3754586123610514, 0.3729939989450314, 0.3755395775581287, 0.3712214451945845, 0.3765020143544961, 0.36880830729519704, 0.37825475155313176, 0.37043180497405853, 0.3724795250545315, 0.37523673915281874, 0.36356267951201665, 0.37091055788258237, 0.3695364404639428, 0.3652442142359063, 0.36200858769413513, 0.36430317647012717, 0.36808979959181576, 0.3550794521600464, 0.0, 0.0, 0.0, 0.0, 0.0, 0.0, 0.0], [0.005874038182803124, 0.010496631455147915, 0.0010671599163470382, 0.007347684029037935, 0.003636579525021486, 0.06764487244511633, 0.1915713499204103, 0.26368292105593355, 0.3343097530264835, 0.36721822846120256, 0.3630726844225369, 0.35824995588104214, 0.3701466201162862, 0.37551044096458547, 0.3797531288201013, 0.36853775818348694, 0.3733232321786994, 0.37544216562693994, 0.3706469490557297, 0.3703845984669406, 0.3795615315245384, 0.3775069728176147, 0.37776387586128096, 0.376606462370514, 0.36695755586002327, 0.37977198718611016, 0.37476274498551027, 0.3767319449347608, 0.3751120274780603, 0.37909506280399774, 0.373587139243338, 0.3776047549170523, 0.3768576021847094, 0.3731974282620911, 0.3776846342927241, 0.36593938245871943, 0.37493915817888, 0.3721048542922282, 0.37017813424231655, 0.3618409833578066, 0.3693004108156233, 0.36622774359394417, 0.3568092375964301, 0.0, 0.0, 0.0, 0.0, 0.0, 0.0, 0.0], [0.008069940407423867, 0.0031474075033902805, 0.003190917883178831, 0.00794411990786531, 0.005624557684818112, 0.07105954783455425, 0.1873757887781817, 0.2602006524486831, 0.3349020826552433, 0.3521161202063123, 0.3709413240804857, 0.3607316764723686, 0.369633453189005, 0.3684659570684785, 0.37838280610582503, 0.37089186977009886, 0.3766134240464156, 0.3785911707886375, 0.36930683943666726, 0.3740397022410094, 0.3822316949868982, 0.37993538885347244, 0.374512510261889, 0.37920096550951166, 0.37215077114384226, 0.3766296110392079, 0.37957318375405424, 0.3764909083946731, 0.3745292437927916, 0.3807858668491329, 0.37569252486956, 0.3799556221612577, 0.3748849868251317, 0.3760154202106018, 0.37786012055689944, 0.37185290992309517, 0.37404372240378025, 0.3716713119393017, 0.37332763171498506, 0.36217628706160204, 0.3685777047737258, 0.3672598138789557, 0.3635180329532452, 0.0, 0.0, 0.0, 0.0, 0.0, 0.0, 0.0], [0.00834933036551048, 0.0035287049957438087, 0.0034564055528880683, 0.0023704516166500288, 0.003484120758869866, 0.08138726338250928, 0.18120940393770738, 0.2642606904074556, 0.3343477967686924, 0.35242227645946744, 0.3626983699470507, 0.3641347753336833, 0.36735772266606903, 0.37385073849106504, 0.37937765473783974, 0.37414244000195407, 0.3769596243443007, 0.3803655213095905, 0.37039816374798323, 0.3730689853436572, 0.38187293013681783, 0.38062874319629747, 0.37808091749039646, 0.3812588840419361, 0.37628054673024947, 0.3821115955453345, 0.37935721997569544, 0.3764988794210725, 0.37638609845475496, 0.3821309829684323, 0.37631630390231857, 0.3775324754573664, 0.3745509600703649, 0.37979513947802185, 0.37842688518895606, 0.3760585314487196, 0.3737797941330939, 0.3748654927564286, 0.3728308295988398, 0.36946629360256295, 0.36662191679934036, 0.3641160347941138, 0.36689595946706716, 0.0, 0.0, 0.0, 0.0, 0.0, 0.0, 0.0], [0.0036360551991227756, 0.003782427575456084, 0.0035232828078007998, 0.004964896875869112, 0.01583425161660456, 0.07903371329325486, 0.17501176017436604, 0.264613649907561, 0.33463337715917, 0.35006480385318284, 0.36608681048530106, 0.35952330466256766, 0.37499236846926115, 0.366249266334612, 0.3758006040862363, 0.3745749983740645, 0.37231505483669264, 0.38379478795419564, 0.37478310917217234, 0.37885827931704424, 0.377997696089872, 0.38042534494231756, 0.37892538545233634, 0.3764242299715274, 0.3768239146314291, 0.3792255691822262, 0.37760654335442706, 0.37804037183658484, 0.3842473464090586, 0.3820494740199425, 0.3765472206048326, 0.38261122585098956, 0.37734958734466484, 0.37898330701199634, 0.3797451886189537, 0.37648117838282025, 0.3760684342360912, 0.37615447197413676, 0.37547753578048626, 0.37535381643427457, 0.37073632189509886, 0.36969024232957043, 0.36638314480537537, 0.0, 0.0, 0.0, 0.0, 0.0, 0.0, 0.0], [0.009809057238385877, 0.005226010604364307, 0.004933584018482133, 0.001955916600078267, 0.006686059617593568, 0.06829278156971957, 0.16740813486989764, 0.2675514029125075, 0.32903996727580886, 0.352930775291943, 0.3650798676672053, 0.36132703097059626, 0.36804150046433165, 0.37318206812258353, 0.37538876527581083, 0.37648360474219755, 0.37282906576385455, 0.3809575076611439, 0.37585883083160077, 0.3825527483386342, 0.37972738027196934, 0.3771906454527105, 0.37643581226531786, 0.3766077521766333, 0.3777472078852682, 0.38146955490500317, 0.3812544073779091, 0.3784466950424741, 0.3760477975597659, 0.38160855336638116, 0.38335781676710884, 0.3771973220753635, 0.3763616391764903, 0.37720863936483573, 0.37482878783245144, 0.37682655155913763, 0.3800918308045188, 0.3775582083080561, 0.36848119170859805, 0.3725889034094632, 0.3734031806385026, 0.3720652957736747, 0.36961456938388043, 0.0, 0.0, 0.0, 0.0, 0.0, 0.0, 0.0], [0.02076076620123751, 0.005660520307606034, 0.007250146191492315, 0.007911364899394084, 0.008483661412432572, 0.08080365716727954, 0.15994704315358085, 0.27093217454169816, 0.33402637970665444, 0.34392526537831275, 0.35992050534534253, 0.36617471586949984, 0.3682635686207703, 0.3743901676748149, 0.378949948864511, 0.37974142052032456, 0.3760068017444336, 0.38062079832947204, 0.3786531104456589, 0.3803986094060733, 0.3773430863897413, 0.37696091052890673, 0.3746392277751826, 0.376996137840018, 0.3801552529317806, 0.38228457297574847, 0.376789134976244, 0.38015010115711245, 0.37739334173452604, 0.3819014628381619, 0.37628997423078747, 0.3836722001537092, 0.37783251514284394, 0.3754286674021289, 0.3775223014833644, 0.37803814893291376, 0.3780977709497747, 0.37757714991324565, 0.3818033641593131, 0.37721116844470437, 0.37570859373489307, 0.37452791811598196, 0.36888564103335214, 0.0, 0.0, 0.0, 0.0, 0.0, 0.0, 0.0], [0.018997063105815674, 0.008645485398732205, 0.0062423906435804455, 0.006678594675777394, 0.009558223208558817, 0.08748218673186198, 0.15103295837555597, 0.2738482232626959, 0.331181387513893, 0.3487615865447135, 0.3556478285345443, 0.36016784002114643, 0.3663037960196287, 0.3736838747945582, 0.37614629933986404, 0.3787919037425408, 0.3812549050474139, 0.3826289164010665, 0.3733661107237438, 0.3797141029887185, 0.37839748652792354, 0.38143934539928986, 0.3753205571319152, 0.38020425376025824, 0.38160464216968204, 0.37870523685976204, 0.3753565061650796, 0.3812824878026765, 0.37705898334433724, 0.38150543395915915, 0.376654658856667, 0.37559108837035965, 0.3724592311254124, 0.38266551402815, 0.37197450430041307, 0.3794253088833369, 0.37931191990211244, 0.37457343796563014, 0.37675774317741517, 0.3756954502803867, 0.37171638264553414, 0.3746072196048799, 0.3741396630590801, 0.0, 0.0, 0.0, 0.0, 0.0, 0.0, 0.0], [0.014736431428194113, 0.012207780531287363, 0.0020537847866437986, 0.00717188090847326, 0.007824801517963097, 0.08848052337085342, 0.14769324389937075, 0.27168382425852816, 0.32874173566829024, 0.34349651560224465, 0.3569609085065816, 0.3652397033874414, 0.36886510294075914, 0.37194826577003, 0.37393639820358937, 0.3765313920974564, 0.3788055543206894, 0.38223382148016566, 0.37293236082053055, 0.37853722770327036, 0.3848211877439927, 0.38822397981045736, 0.37847586307011144, 0.38092703264829997, 0.3800704567835992, 0.37508035019764724, 0.37258654824790816, 0.377080425282902, 0.38184303513901136, 0.3816976360515758, 0.377968642000518, 0.3880142120792881, 0.37293386676631574, 0.3747938377026797, 0.3764146248588833, 0.37883453768726616, 0.37648289832353543, 0.37202113332538916, 0.37599314348564833, 0.37082164485872343, 0.3749950994290321, 0.37434373158585876, 0.3700377199663054, 0.0, 0.0, 0.0, 0.0, 0.0, 0.0, 0.0], [0.014063982379760859, 0.010329132788545307, 0.006312350005967617, 0.006326628439704306, 0.010211220816776305, 0.08818212248274823, 0.14281112099698245, 0.2700201952928974, 0.33107305372170875, 0.339954042882778, 0.36088206809045636, 0.36407499124477666, 0.37093028143367235, 0.3697795035241366, 0.3783928674231371, 0.37206495922766014, 0.37541332398116944, 0.3812444321681196, 0.37603322860023636, 0.37435514155782484, 0.37730875982909157, 0.3822138419462677, 0.380577530766477, 0.38116565136182157, 0.38027593789099473, 0.376673666984871, 0.37158693231502743, 0.3809554226926662, 0.37607601618403036, 0.38492054658919556, 0.3745111658344393, 0.38249128675921557, 0.3738832294919595, 0.37366243347887157, 0.3738742848973615, 0.37419097572687543, 0.3772394400901773, 0.3717474289304418, 0.3748973517945019, 0.3705468109427555, 0.3759114391276763, 0.3722764424510804, 0.3727098564141306, 0.0, 0.0, 0.0, 0.0, 0.0, 0.0, 0.0], [0.018795810079558214, 0.009507011480333501, 0.01035843132055787, 0.004880372064203893, 0.009529895911583118, 0.08999983040862644, 0.14150572280873644, 0.27292886871244826, 0.331383265645708, 0.33212118227113435, 0.3639177681109861, 0.3663518775962441, 0.3708453204932739, 0.37489806079933924, 0.38144500729560205, 0.3760544855879575, 0.3750769513509879, 0.3722952554975402, 0.3796363839285287, 0.3711384911119795, 0.37689857306639696, 0.3777518538239802, 0.3800070197066784, 0.38184017014543986, 0.3847274911932113, 0.3792047552974402, 0.37560709155830607, 0.37630924820043865, 0.37709648267569723, 0.38637162584453316, 0.3812542141719924, 0.3839700892273426, 0.37432531995364493, 0.3747906290307064, 0.37293446083568577, 0.3743790843298727, 0.37757560318643757, 0.37280360198428847, 0.3745891401359501, 0.3750457835142561, 0.37599181430627354, 0.37514091890213164, 0.37390571327476313, 0.0, 0.0, 0.0, 0.0, 0.0, 0.0, 0.0], [0.019524099814536906, 0.00671648692723867, 0.008194005195530983, 0.005129482383530752, 0.01600801670738418, 0.08915545508532788, 0.14139229093029573, 0.27471780882574315, 0.32919187341291295, 0.3376695943698526, 0.3589073382081811, 0.3669153618989552, 0.3737542513225043, 0.37347204302090914, 0.3807778455344981, 0.37564683586843484, 0.38094007087156845, 0.37791881011865636, 0.3793820459757648, 0.3758466019892393, 0.37532156191108734, 0.379415558318946, 0.3760260901961436, 0.38329610675026665, 0.38469588381989517, 0.38352914871606725, 0.37492394578250665, 0.3779223208402726, 0.37645597166589334, 0.3822206498990719, 0.38010941651279956, 0.38300920798882454, 0.3756298769575073, 0.3719354501202113, 0.3725966767071647, 0.37650558212913393, 0.3737738894552983, 0.37533760852451703, 0.37567005664214365, 0.37541547710773254, 0.3733151676054471, 0.37750271924334916, 0.36772177283019947, 0.0, 0.0, 0.0, 0.0, 0.0, 0.0, 0.0], [0.022576777220459407, 0.0010665136040384333, 0.00961705456454593, 0.00564596460467967, 0.01516310434334482, 0.0998349314503234, 0.1451941884252245, 0.27695395274438445, 0.32870527539163336, 0.3442717019648297, 0.36077541761090126, 0.3601770956303978, 0.3717352510161739, 0.3677750719160778, 0.3845738276091659, 0.37116468687052084, 0.3770166876178943, 0.3775680278135582, 0.37478605750407884, 0.3801262272740895, 0.3820935595896898, 0.3763603332161693, 0.3781261673747773, 0.37370066222730636, 0.36152811444424426, 0.38651201256027923, 0.37512825122828464, 0.3780511549286837, 0.38151991018745923, 0.37999794897412376, 0.3792734609183436, 0.3816212805472886, 0.376642479109276, 0.3740602732742185, 0.37285898445706805, 0.37442048039985204, 0.37623436930109283, 0.3720674056238753, 0.3755336394516991, 0.37910916821554547, 0.37316987378101996, 0.3774751524207678, 0.37267055014749634, 0.0, 0.0, 0.0, 0.0, 0.0, 0.0, 0.0], [0.014403860830615062, 0.009409112017126426, 0.010437104954631272, 0.004709560436543957, 0.009791110657557412, 0.1025014282884444, 0.1451487987316608, 0.2751357591084218, 0.32827321045443153, 0.34207996783819733, 0.3637041756485884, 0.35987151884949736, 0.3672705861726116, 0.3692228145927751, 0.3751401271599483, 0.3682773876071658, 0.3729735800039694, 0.38101193854814447, 0.37715636713639583, 0.3759023567049589, 0.3814810875459524, 0.3794765626323808, 0.37581628764643077, 0.3630924243439549, 0.21061286866829337, 0.3771817329423378, 0.37943503431908243, 0.37565297341149223, 0.3806423453488142, 0.3804472609390342, 0.3825851019363978, 0.38733661627558097, 0.37496362414870726, 0.3754924192534808, 0.3717128999146145, 0.3695127405566593, 0.3761855031799551, 0.37379570186977334, 0.3763229995660998, 0.3776707744806504, 0.37843888370537704, 0.37441336856308777, 0.3732610659551286, 0.0, 0.0, 0.0, 0.0, 0.0, 0.0, 0.0], [0.012190321079227061, 0.0070428003271937505, 0.005023422515498981, 0.009151871489915054, 0.017214094193941792, 0.11368552928458546, 0.14335150044941317, 0.2745339540794717, 0.3244493196913974, 0.34010664809893987, 0.361970257406158, 0.36103293819613913, 0.365309866553671, 0.3683379770790713, 0.3717863960353691, 0.37017765400128366, 0.3709003500978061, 0.38129183807495515, 0.3732183888816341, 0.37950947727169576, 0.37766533583460277, 0.380176819042097, 0.3833165386970541, 0.37654325514122183, 0.37425707678297393, 0.3769403489754662, 0.3852408930820819, 0.37542781905167644, 0.37842838642454435, 0.38484228146375477, 0.37907517793550716, 0.38478579405316965, 0.3788337105857005, 0.37682196122172856, 0.37737301842808424, 0.375854462148075, 0.3797430654665444, 0.3735830014429939, 0.3784523043200123, 0.38183045322415027, 0.38380502398523547, 0.37700355085990017, 0.37732829143394175, 0.0, 0.0, 0.0, 0.0, 0.0, 0.0, 0.0], [0.014961408589921203, 0.005212396531106415, 0.00833471844152925, 0.007295368167710498, 0.008599417618132606, 0.09935187803324087, 0.14417162444547746, 0.2745257583623179, 0.3245449218620534, 0.3430875093270893, 0.3594743521461139, 0.3594549663180187, 0.36539748086388313, 0.36684369526229327, 0.3716545905334834, 0.3717078510723937, 0.37403437417309765, 0.37498408488642315, 0.37265909167445815, 0.3770345047258428, 0.3764699785170958, 0.3793542286323397, 0.37868466060129347, 0.3815077390546621, 0.37989389489531056, 0.3708060468980512, 0.37507180692553144, 0.3778490326658219, 0.3831824357879161, 0.3831840325739631, 0.38151954795890225, 0.3801483603412471, 0.37776038811420665, 0.3810971571443963, 0.3788117275664848, 0.3766746102804423, 0.3824227724814226, 0.3752301082180802, 0.381669716307544, 0.38002721238478887, 0.37898613459395986, 0.3776977586556069, 0.3786294974541298, 0.0, 0.0, 0.0, 0.0, 0.0, 0.0, 0.0], [0.013819335201515962, 0.011977242495173934, 0.007433199020602398, 0.0046064101499468995, 0.013773605716967688, 0.10922709709846691, 0.1544759869744373, 0.283825251783376, 0.3260733962144033, 0.3468982706936419, 0.3593960241666959, 0.3605350115996475, 0.369963018141718, 0.3642990868459405, 0.3739338387728186, 0.37629722392944875, 0.38153092816998585, 0.3758062465876359, 0.37337517642228074, 0.3819733290790851, 0.38106678790493137, 0.38003283391622616, 0.3838718663030416, 0.37569289561146524, 0.38498638971826427, 0.37892628183435295, 0.377129652339344, 0.37650516239545484, 0.3851825815200494, 0.38113116257000784, 0.37956399229090565, 0.3832022756242576, 0.3809924264025236, 0.3802917271852268, 0.38627324656830686, 0.3827030634543836, 0.3802101731403301, 0.3773178686063527, 0.38278158202790075, 0.3820230008320901, 0.3827453309018563, 0.38003467070339475, 0.37306420957788694, 0.0, 0.0, 0.0, 0.0, 0.0, 0.0, 0.0], [0.010480611249860048, 0.008016958261760382, 0.004671080715239213, 0.010645553169799322, 0.012405829540016186, 0.11918341015243311, 0.17449793720184675, 0.28248871585708735, 0.33279460823941964, 0.3470175275505428, 0.3657355549942788, 0.36388281572463765, 0.3728759877778429, 0.3703578792891596, 0.38127166589749967, 0.382743789104023, 0.3836260117525597, 0.3795919354361731, 0.3802857506943009, 0.3845832098765035, 0.38237514611197193, 0.38662443487389714, 0.38334302611048077, 0.3840895159209107, 0.38793212724921877, 0.39396018518757936, 0.3792716696116383, 0.37715239538901396, 0.38531088436098243, 0.3893005930293196, 0.3848977877510692, 0.380767469436278, 0.38308589142628585, 0.38467911436963864, 0.38237811346276307, 0.3896442086481701, 0.3849957818764917, 0.38310750438633684, 0.3873793799553634, 0.38779172357387975, 0.3878092111134974, 0.3858039801346766, 0.3849804670784357, 0.0, 0.0, 0.0, 0.0, 0.0, 0.0, 0.0], [0.00837501781777275, 0.010224101071703821, 0.0022798820503251785, 0.0048157743306537415, 0.007349701045394087, 0.1313054231143284, 0.19976743442375836, 0.29169204338885496, 0.3364264099623392, 0.35935054729575305, 0.3708195231413906, 0.3716603487703452, 0.37357280351248917, 0.37813611745313236, 0.38670613406728566, 0.38421846327736053, 0.38213403495918236, 0.3843302952206057, 0.3858422982660456, 0.38922470077104393, 0.3901623429347446, 0.39086015762420334, 0.38809369464093474, 0.3888176506880536, 0.39314553543214875, 0.39436715170704645, 0.40030820204714834, 0.3853093874758702, 0.3906720019612236, 0.3897532498643701, 0.3954421066927805, 0.4009744712743751, 0.3824371674541337, 0.3933836207646004, 0.3906381215449711, 0.38920163696815585, 0.3914459863380308, 0.3861915804252514, 0.38968296985032636, 0.39179613915440936, 0.3989775128496451, 0.3938875725320584, 0.3864974900472333, 0.0, 0.0, 0.0, 0.0, 0.0, 0.0, 0.0], [0.00838877532520911, 0.010589914879949059, 0.002224042531040736, 0.006106079443469093, 0.017926193039910127, 0.14069251871568444, 0.2307339319918316, 0.3082585362899542, 0.34994421870735143, 0.37508174225159635, 0.38164065910167905, 0.38671353514454565, 0.3845385748947001, 0.3903698866967733, 0.39477105168397536, 0.3947910647559805, 0.3928794966599405, 0.3895095028488699, 0.39134332461513444, 0.39743060053665774, 0.3983950492389707, 0.3996286225985688, 0.39591217106366816, 0.3963523230697301, 0.39821788072215086, 0.4027626585942604, 0.40076471352228143, 0.41034075177858753, 0.3994034247343273, 0.3982458407860563, 0.3966656075110676, 0.41095646758236515, 0.32568776202884164, 0.3949969186821802, 0.390594328392621, 0.3978373500125515, 0.4000227513471393, 0.39519499687033766, 0.3928977463305613, 0.40026604325119164, 0.3976832477713285, 0.39892739651412373, 0.39837066977457153, 0.0, 0.0, 0.0, 0.0, 0.0, 0.0, 0.0], [0.008427427126380503, 0.010857270776764372, 0.0017473895369396412, 0.00920217068151753, 0.018226008474598314, 0.14365265913127076, 0.2656622544396674, 0.3291565361073264, 0.3664156565394767, 0.3878731865505964, 0.39694920078654555, 0.3977237892544911, 0.3993359460308425, 0.40223076035516575, 0.40507782471819537, 0.40577060871224374, 0.402998042891559, 0.4010182848821386, 0.40341009554491025, 0.40698576023223226, 0.4104783317070037, 0.40750804257896045, 0.4076770430225669, 0.40543102289879435, 0.4091436105736839, 0.4106413746221875, 0.4116859927466865, 0.41218829941098156, 0.4235580981717647, 0.40943625570641423, 0.40626387602348757, 0.40896999889612895, 0.36847889508461534, 0.3901319973171126, 0.4046054625408445, 0.408275084913178, 0.4129337375091648, 0.4044431317190332, 0.4019334492870749, 0.41378827760940423, 0.40793173164382807, 0.40934378448034564, 0.41124454748824685, 0.0, 0.0, 0.0, 0.0, 0.0, 0.0, 0.0], [0.010697979980577376, 0.006382974982283756, 0.005007395716848267, 0.00616668846927355, 0.016922476981168152, 0.14976094367558873, 0.3069306767874662, 0.356818928272043, 0.38448383850681955, 0.39761913978386065, 0.40867651038664266, 0.41068759025705426, 0.4083566449572175, 0.41668591078267025, 0.4214535124989155, 0.4228664848131796, 0.41784993902054396, 0.41657820594062767, 0.4189663275171555, 0.41906870921470685, 0.4206069124007058, 0.4163484360690146, 0.4199623241242405, 0.41758474895577186, 0.42372719813958315, 0.4228102862002592, 0.4171320276018279, 0.42543164851462273, 0.4277816164423132, 0.44214649288519053, 0.42486242811961533, 0.42286901339063004, 0.42173022107245683, 0.43070874884720856, 0.42721864043846586, 0.4262512332487706, 0.42723991083295515, 0.41806897856703257, 0.4134247094690971, 0.4218526382381931, 0.41519700556377775, 0.42164978347626103, 0.4180339424106401, 0.0, 0.0, 0.0, 0.0, 0.0, 0.0, 0.0], [0.01063519211076513, 0.008692379327867051, 0.007392558205328696, 0.0038478980633045654, 0.01867617619344138, 0.15683141575701065, 0.340913203559503, 0.3894189046702048, 0.3955034539998628, 0.40610961169907445, 0.4142483280749874, 0.4092344433450037, 0.41321395767286845, 0.4249714380506677, 0.426328102612725, 0.4215554761267998, 0.4243174444074896, 0.4198317098542801, 0.4234709706100903, 0.42544171545670956, 0.4318881905827074, 0.4224694220362657, 0.42834318070679245, 0.42534247728855246, 0.4332276890600195, 0.43827528309130825, 0.4292606228166839, 0.4282688986614821, 0.4348023862212428, 0.4433005385927758, 0.4561720459376776, 0.441907668955597, 0.4285648936504218, 0.42769040328982333, 0.44843907487270696, 0.4551501341628969, 0.45501882737800436, 0.4451228354103719, 0.43180258978429786, 0.4316467742220851, 0.4282980677104874, 0.4306950531524574, 0.4226415105399983, 0.0, 0.0, 0.0, 0.0, 0.0, 0.0, 0.0], [0.014980833179335313, 0.012186501734011571, 0.005195056037650901, 0.007379705549340375, 0.028746597233235926, 0.18407407713853652, 0.34565177786273704, 0.40924919197592596, 0.3943816268015037, 0.3831585956476476, 0.3770575073997884, 0.33627494882072234, 0.35921041235827594, 0.3796689061976934, 0.3767645657323931, 0.38133898551006157, 0.37955188252860256, 0.3735386348483489, 0.3487547784676358, 0.3801376392203985, 0.37984862212811804, 0.3876112347338837, 0.3908083139855385, 0.3789094303868777, 0.3850361814796707, 0.3927397158005936, 0.39107275423890775, 0.40004206754084226, 0.3938651221559171, 0.4030002020103977, 0.41490409153255875, 0.434848434262212, 0.40764383244626107, 0.40229506248033425, 0.39774532575428895, 0.42332888268686886, 0.43911867119303566, 0.4342382095802811, 0.4287920884217159, 0.4257925801530649, 0.4244963483565999, 0.4159490171486222, 0.0, 0.0, 0.0, 0.0, 0.0, 0.0, 0.0, 0.0], [0.008035020738601836, 0.009738882867923295, 0.007253915636661449, 0.007717688967355979, 0.013095006246848138, 0.13140394495755434, 0.24465516632767603, 0.29057320172114554, 0.26183336398685775, 0.24889467168530446, 0.23804482376969427, 0.20918263008300084, 0.13989735781762924, 0.24104996644857382, 0.23616325732413848, 0.24564230425428038, 0.23831591293845586, 0.24607147950247274, 0.2376567368661888, 0.25569669713880283, 0.24238148523232977, 0.2566933199670111, 0.2671028951813216, 0.2656689276424794, 0.2710194259772214, 0.2628947747026879, 0.27585595779418376, 0.2774431856753411, 0.27584412080915593, 0.29214063673137125, 0.28838704666431936, 0.3018166545558153, 0.30555580368309787, 0.2956692704123688, 0.28366257723533894, 0.2885270026898204, 0.3143412300750751, 0.31329737721016476, 0.323354485706713, 0.3105664749436856, 0.3073696911644936, 0.2989495704163188, 0.0, 0.0, 0.0, 0.0, 0.0, 0.0, 0.0, 0.0], [0.007243073566176408, 0.004553429095571829, 0.0024245832284434444, 0.004672524394776943, 0.00665229532401032, 0.06498962551353271, 0.16919390641721752, 0.13606150478639567, 0.11328998206008976, 0.09991863905512693, 0.09518161406407726, 0.09364794385687318, 0.06379136281275542, 0.09262996541597474, 0.10160033133861764, 0.1068684503028359, 0.10591804771022396, 0.11111038054992427, 0.10736933543466956, 0.1175646637845341, 0.11804046819570227, 0.12009484087200899, 0.12104913998200867, 0.12305904048402803, 0.12630893285979522, 0.12969856910004218, 0.12914837919418645, 0.13263776081006146, 0.13547466439009692, 0.13308841260758875, 0.14646856648862439, 0.14842238177827746, 0.15180107269884263, 0.15332069193193829, 0.16256379043269376, 0.15508049636100435, 0.15393276640639875, 0.1620237485243436, 0.16831654570637655, 0.17196506333953776, 0.16310068867933525, 0.16718759684819312, 0.0, 0.0, 0.0, 0.0, 0.0, 0.0, 0.0, 0.0], [0.0025912666708181506, 0.0016889678771434672, 0.0025973719793630405, 0.007658971186638646, 0.010083791905167007, 0.005353732926402443, 0.0035523664085177265, 0.0033687314794792742, 0.00427202476505395, 0.006183820110149402, 0.00826283771321159, 0.010198741756207576, 0.0070285173250105755, 0.01825089980183198, 0.01630938999827764, 0.016700667325138422, 0.009830052698747361, 0.006844957055921588, 0.0036944424737397953, 0.004917342029499335, 0.0053956717175283634, 0.0041736854773201815, 0.005478915261327197, 0.005225682940877396, 0.007993645870540876, 0.007173217802147092, 0.005271257663477602, 0.003190075678794731, 0.009893521812243155, 0.014394994661743283, 0.004730938397644923, 0.0035816872670799025, 0.004384084907721078, 0.007128827406780481, 0.009415018327407723, 0.008862864846866965, 0.011343839987921805, 0.007967473189661801, 0.004873255906625393, 0.01994398876975432, 0.005120065574004007, 0.008278703393326788, 0.0, 0.0, 0.0, 0.0, 0.0, 0.0, 0.0, 0.0], [0.0033757441676194274, 0.002529765156297227, 0.001983185533032294, 0.005757316982145688, 0.007755449702393323, 0.004679527237199694, 0.0017027880349693271, 0.0022245657801544423, 0.0034134534470581044, 0.0066641743602073485, 0.009370289747214905, 0.007278876274604751, 0.00725460942177942, 0.009651305081525443, 0.013414995366497005, 0.014438169482370661, 0.011419487165713251, 0.006257131860028528, 0.0018983846822765316, 0.005119939926849242, 0.00801617667879538, 0.009540169764140122, 0.0034966339959355552, 0.00043871428849990825, 0.004599944122761372, 0.00041881021430395445, 0.0022730477431398767, 0.00478979172120599, 0.0016109539273659302, 0.008456754276415273, 0.011050405531529979, 0.004393601955324342, 0.005877529369894579, 0.009479827766823911, 0.008925864158403013, 0.005591877927907333, 0.004006100891784472, 0.0018487855462937096, 0.007929919064921902, 0.014972003260567432, 0.0005561387963836224, 0.00879457850728093, 0.0, 0.0, 0.0, 0.0, 0.0, 0.0, 0.0, 0.0], [0.003869957164367688, 0.004097054395851347, 0.004579681632775851, 0.006691685620464892, 0.004360288028740374, 0.0032273067813187242, 0.001770338706812025, 0.0035436022937912343, 0.0010651771081696074, 0.005560522106743287, 0.00883939265974741, 0.005983231540720665, 0.006656376928034706, 0.007307719337193793, 0.011148276893755677, 0.012085992587196651, 0.009594182019653638, 0.006578507951204253, 0.005498583383737611, 0.003836160569656549, 0.009898689833194323, 0.004371627209238786, 0.003183778812164033, 0.0017457879718139333, 0.0038823053329247047, 0.0056881066834598495, 0.004444928528276825, 0.003020251507985131, 0.004799844452393842, 0.004031916274628987, 0.01215347798552671, 0.008277620883087602, 0.005497116658573516, 0.009184069525870465, 0.005725312773285955, 0.0037220076801095935, 0.0008744098441942013, 0.0025208580434124836, 0.009374847282542842, 0.00546457742844689, 0.008360681594207692, 0.006788118381380435, 0.0, 0.0, 0.0, 0.0, 0.0, 0.0, 0.0, 0.0]]
  in  "Integration time (s)":dbl=0.05
  in  "?":bool
  in  "?":bool
  in  "Halt program":bool=TRUE
  in  "Step Size X (um)":sgl=30.0 format="%.8f"
  in  "SerialNumber X":string="70283584"
  in  "Step Size Y (um)":sgl=30.0 format="%.8f"
  in  "SerialNumber Y":string="70283584"
  # "** notice that these aren't\nkcube steppers --> do they still\nwork with the subVI?"
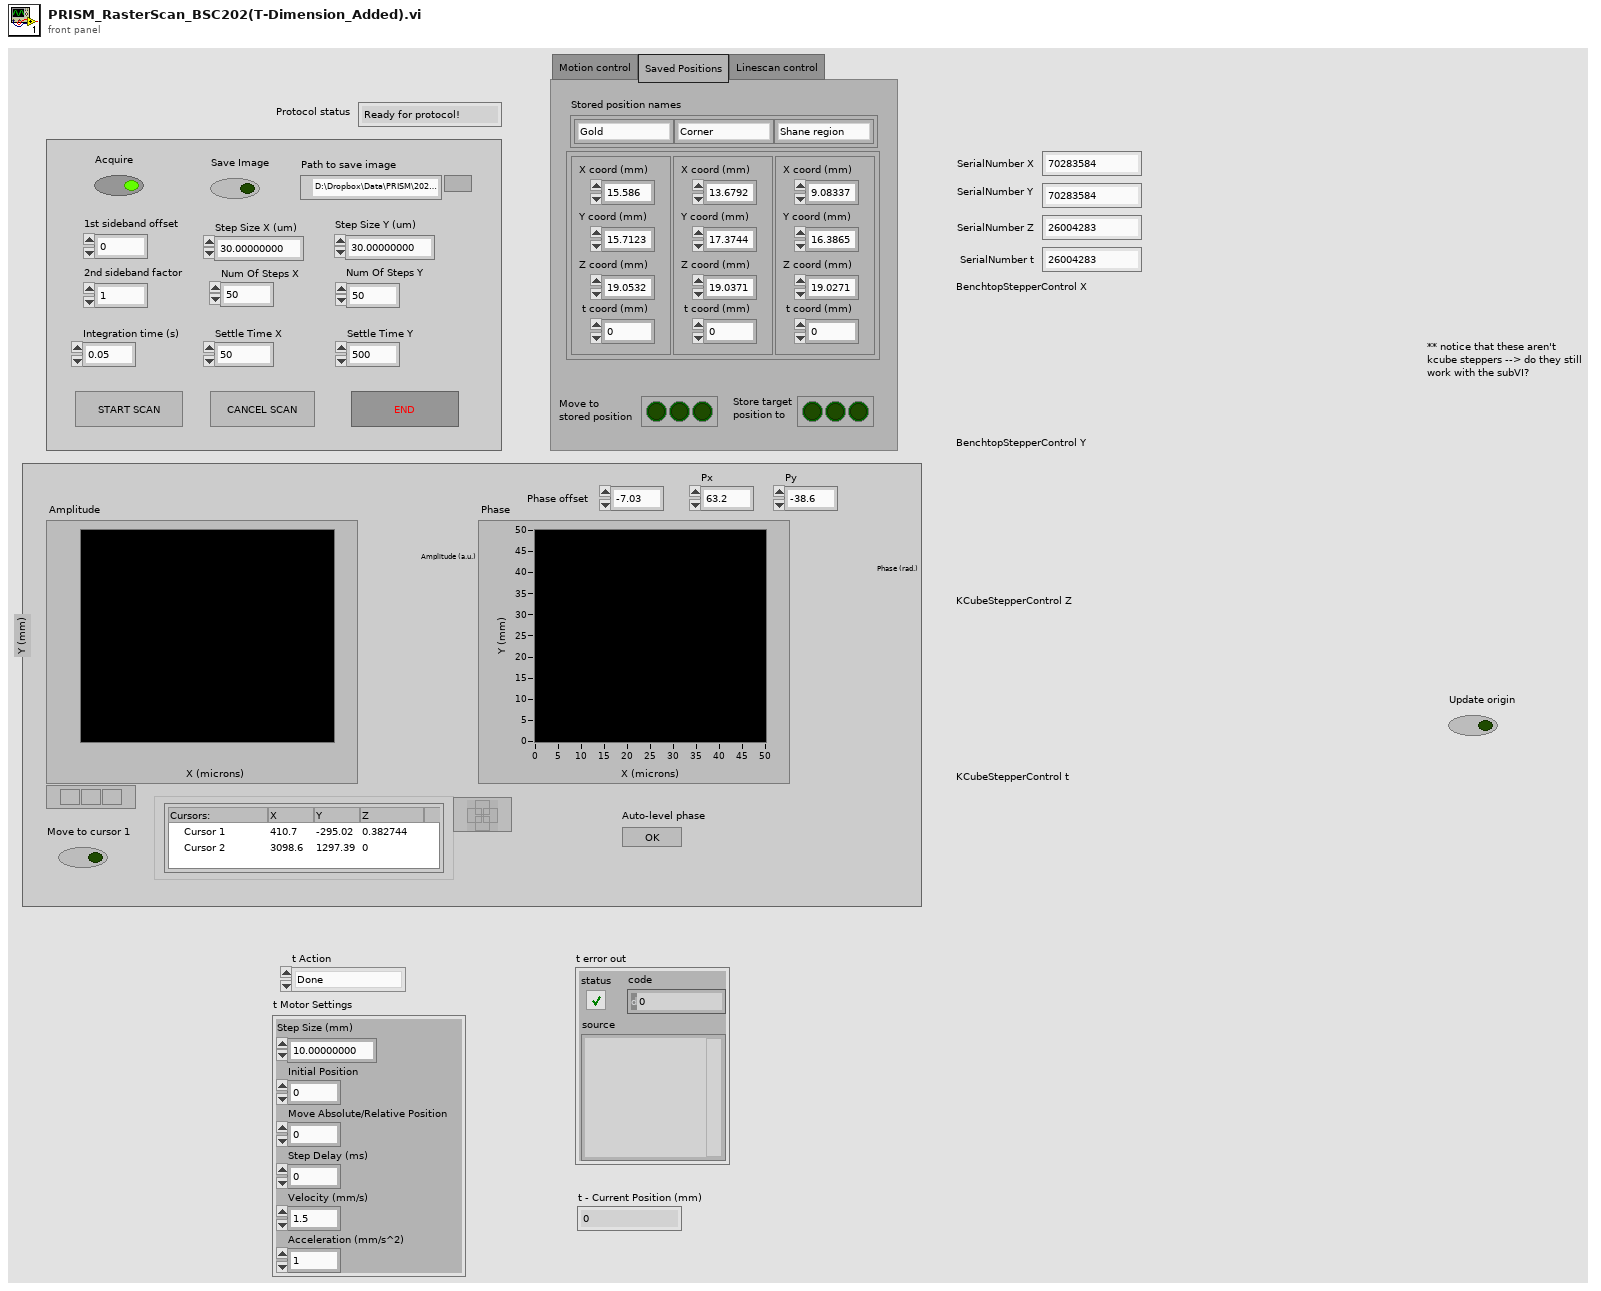
[diagram p1: front panel]
types:
  T1 = typedef "ActionEngineEnum.ctl" = enum16{"Open Connection", "Done", "Get Position", "Settings", "Home", "Move Absolute", "Move Relative", "Step", "Close Connection"}
  T2 = cluster{"Step Size (mm)":sgl, "Initial Position":dbl, "Move Absolute/Relative Position":dbl, "Step Delay (ms)":u32, "Velocity (mm/s)":dbl, "Acceleration (mm/s^2)":dbl}
  T3 = enum32{"Motion control", "Saved Positions", "Linescan control"}
  T4 = cluster{"X coord (mm)":dbl, "Y coord (mm)":dbl, "Z coord (mm)":dbl, "t coord (mm)":dbl}
  T5 = cluster{"X coord (mm)":dbl, "Y coord (mm)":dbl, "Z coord (mm)":dbl, "t coord (mm)":dbl}[]
  T6 = typedef "Control_PRISMRasterScan_ProtocolsLoop.ctl" = enum16{"Sit Idle", "Generate linescan points", "Initialize Linescan", "Update Linescan target", "Move linescan and wait", "Finalize linescan", "Move to stored position", "Store target position"}
  T7 = typedef "Control_PRISMRasterScan_ActivityLoop.ctl" = enum16{"Sit Idle", "Move to target", "Update origin or target position", "Move to origin"}
  T8 = typedef "Control_LineScanCounterAE.ctl" = enum16{"Initialize", "Activate", "Attach indicators", "Increment Point", "Query", "Do Finish Point", "Acknowledge line", "Deactivate"}
  T9 = cluster{dbl, dbl, "Z coord (mm)":dbl, "t coord (mm)":dbl}
  T10 = typedef "LVCursorListTypeDef.ctl" = cluster{"Name":string, "Color":u32, "Style":u8, "Point Style":u8, "Name Visible":bool, "Allow Drag":bool, "Cursor Mode":u32, "Plot":i32, "Index":i32, "Position":cluster{"X":dbl, "Y":dbl}, "X Scale":u32, "Y Scale":u32, "Watch Plots":i32[], "Watch All Plots":bool, "Plot Area":i32, "Label Offset":cluster{"X":dbl, "Y":dbl}}[]
  T11 = cluster{"Name":string, "Color":u32, "Style":u8, "Point Style":u8, "Name Visible":bool, "Allow Drag":bool, "Cursor Mode":u32, "Plot":i32, "Index":i32, "Position":cluster{"X":dbl, "Y":dbl}, "X Scale":u32, "Y Scale":u32, "Watch Plots":i32[], "Watch All Plots":bool, "Plot Area":i32, "Label Offset":cluster{"X":dbl, "Y":dbl}}
  T12 = typedef "imagedata.ctl" = cluster{"image type":i32, "image depth":i32, "image":u8[], "mask":u8[], "colors":u32[], "Rectangle":cluster{"left":i16, "top":i16, "right":i16, "bottom":i16}}
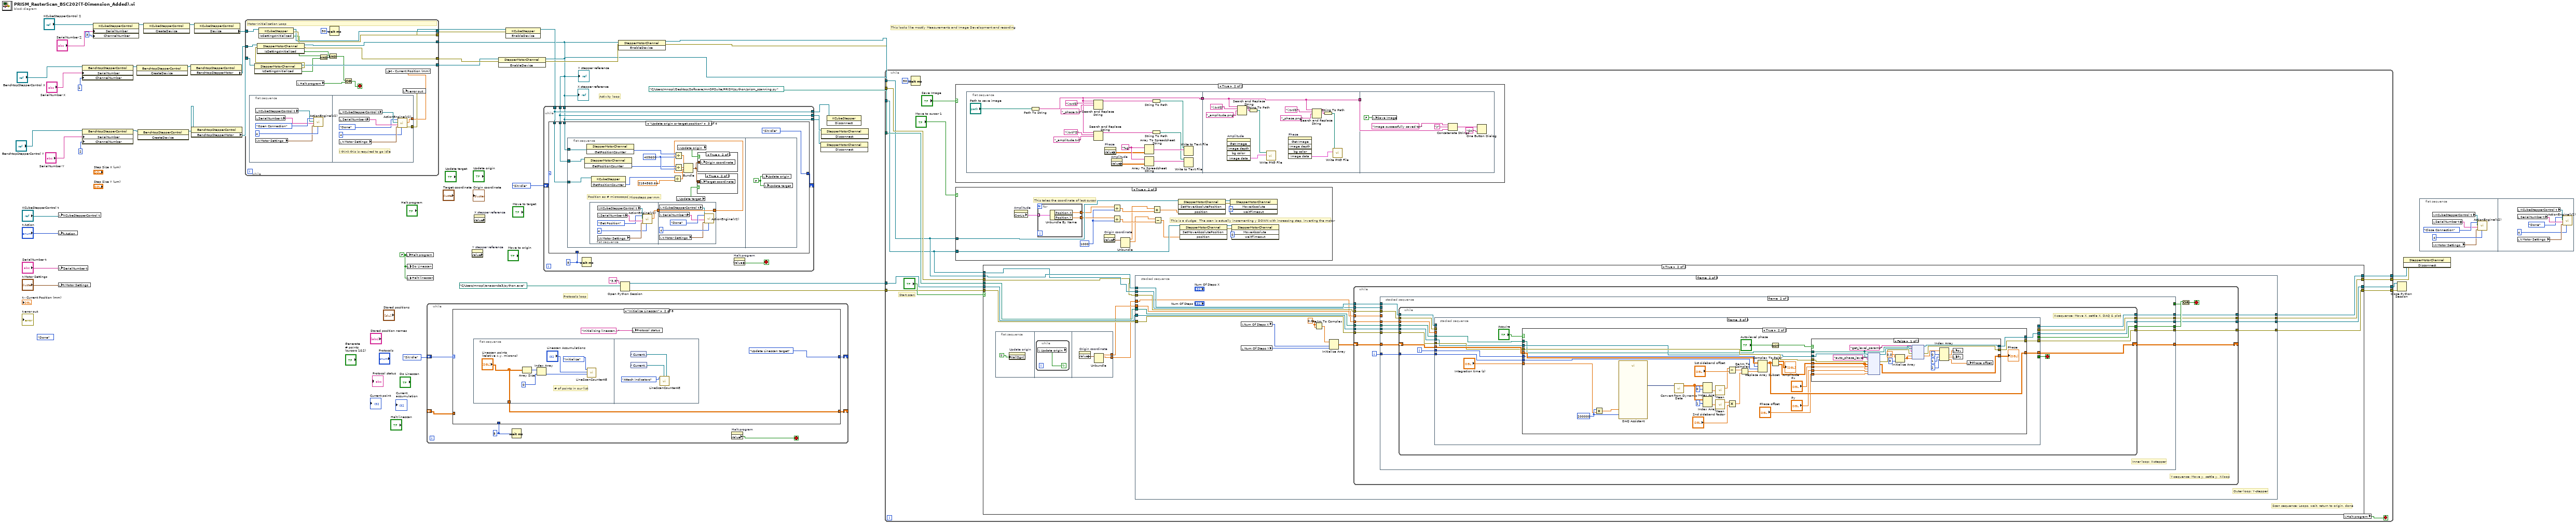
[diagram p0: block diagram]
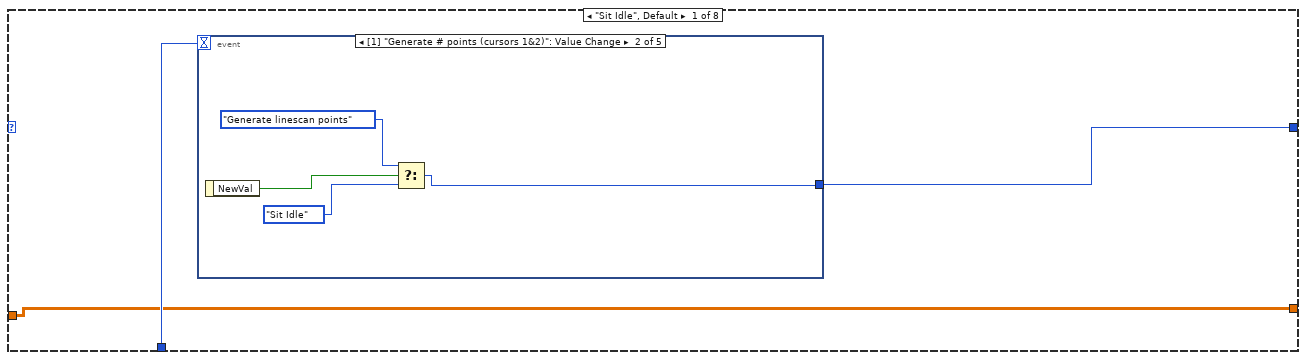
[diagram p2: hidden frame]
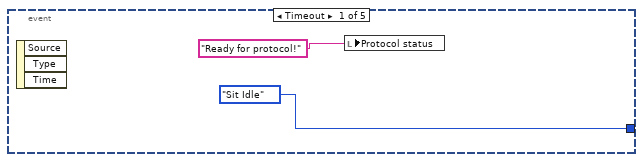
[diagram p3: hidden frame]
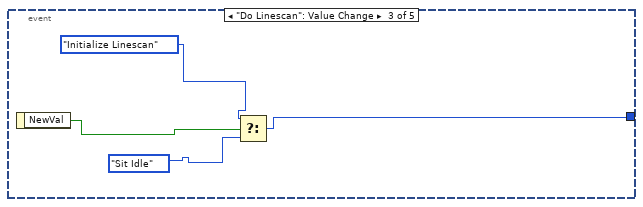
[diagram p4: hidden frame]
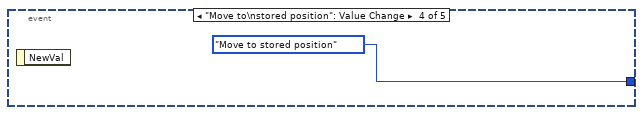
[diagram p5: hidden frame]
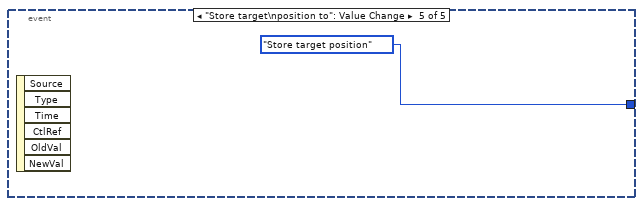
[diagram p6: hidden frame]
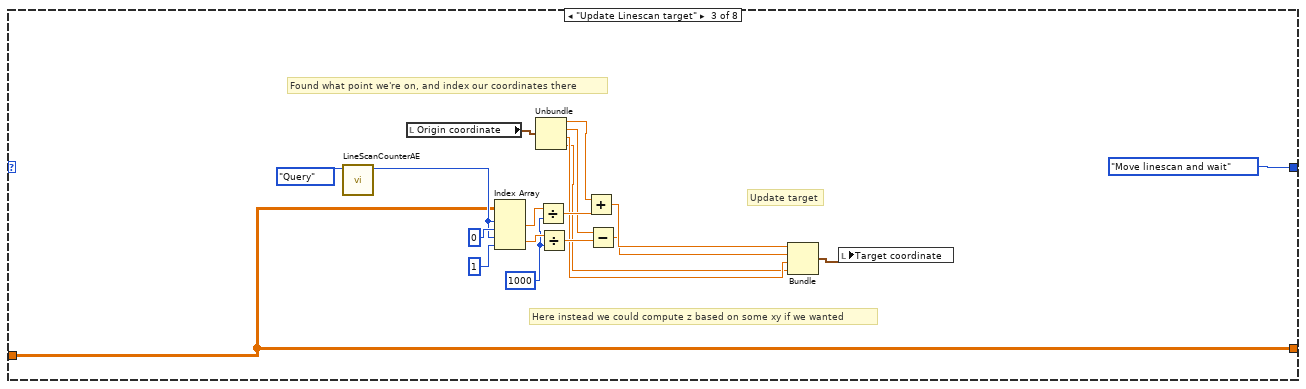
[diagram p7: hidden frame]
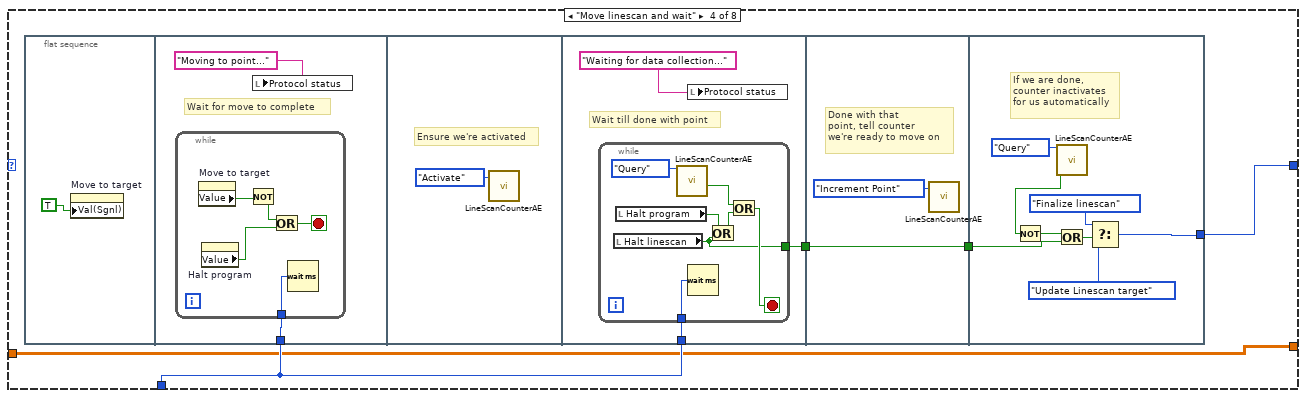
[diagram p8: hidden frame]
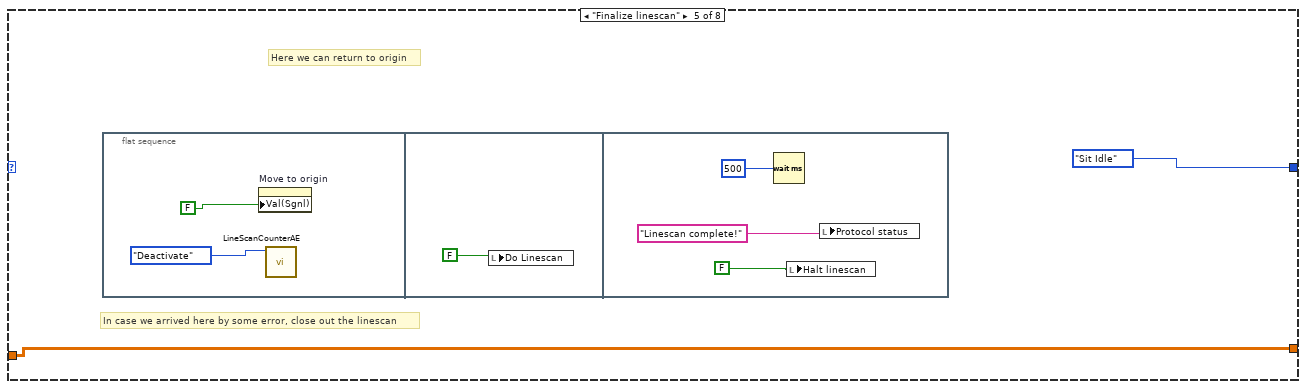
[diagram p9: hidden frame]
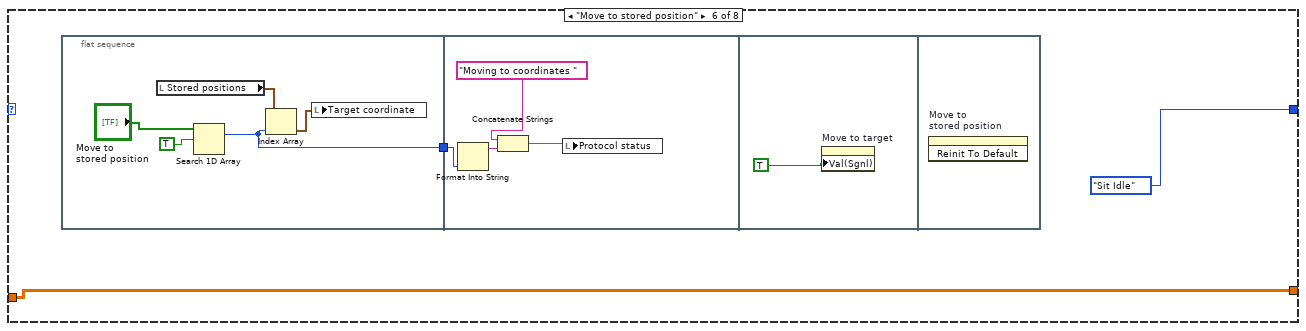
[diagram p10: hidden frame]
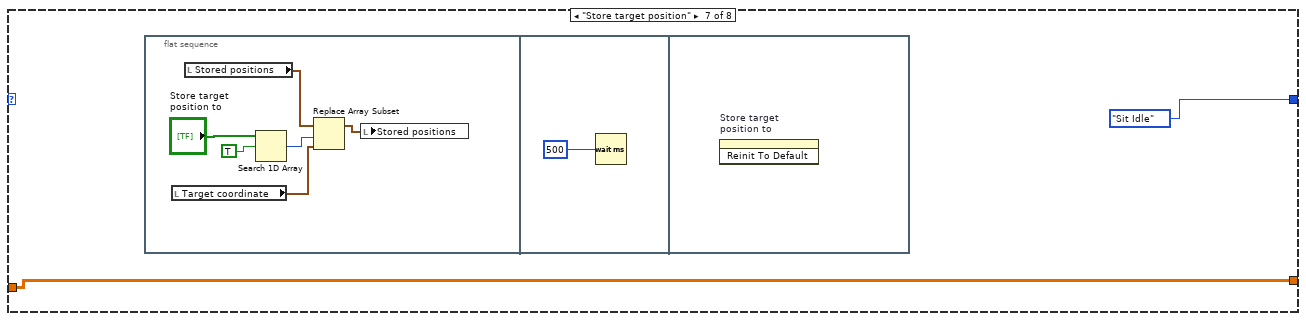
[diagram p11: hidden frame]
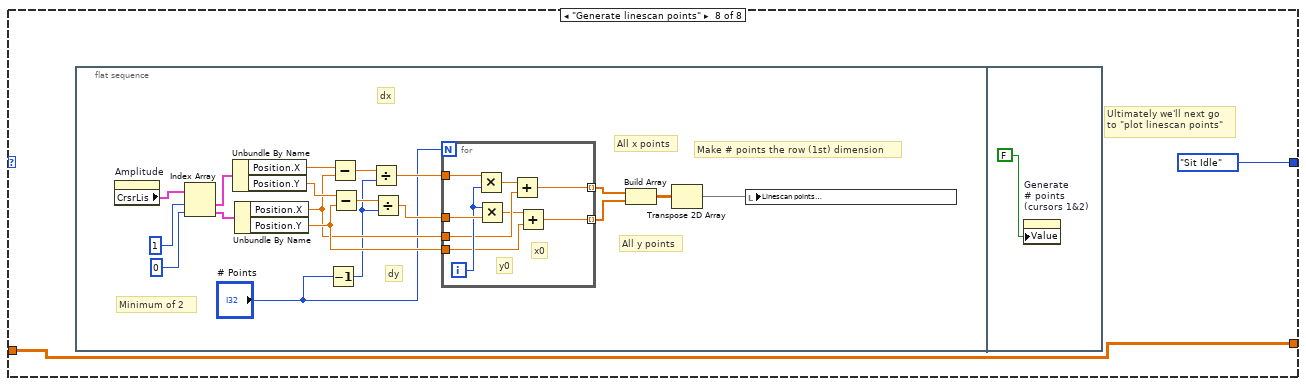
[diagram p12: hidden frame]
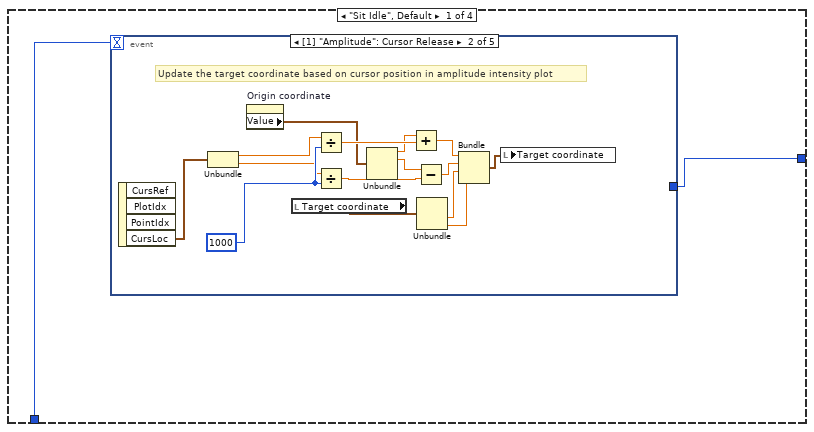
[diagram p13: hidden frame]
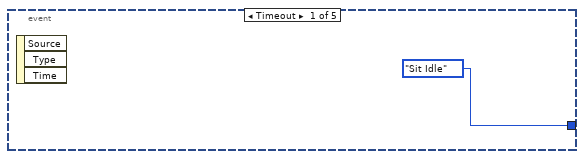
[diagram p14: hidden frame]
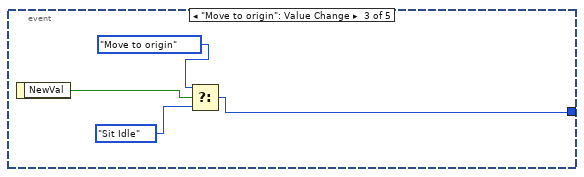
[diagram p15: hidden frame]
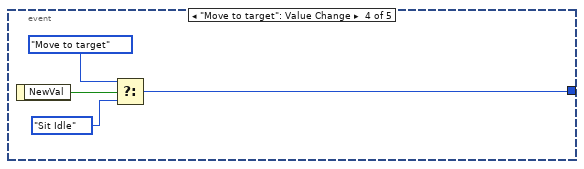
[diagram p16: hidden frame]
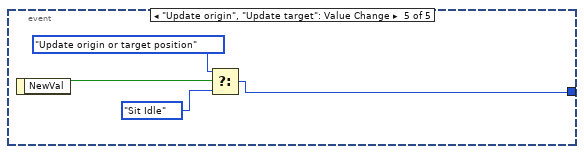
[diagram p17: hidden frame]
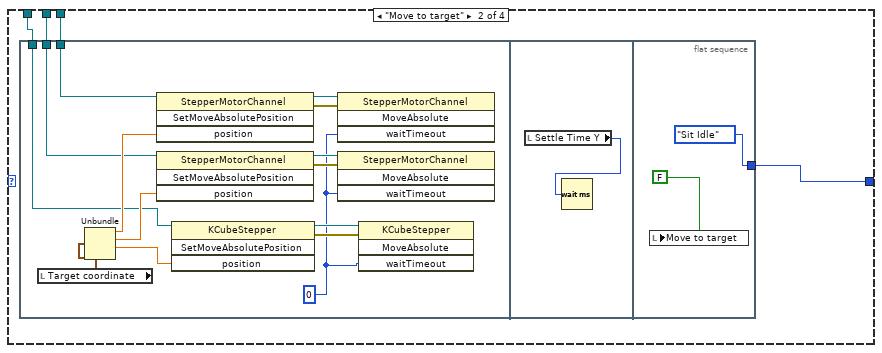
[diagram p18: hidden frame]
diagram:
  (unwired) ActionEngineEnum."Done" ("Action")
  w11 = FALSE
  # "This looks like mostly Measurements and Image Development and recording"
  # "Protocols loop"
  # "Activity loop"
  n1 = local write "KCubeStepperControl t"("KCubeStepperControl t") -> ()
  n2 = local write "t Action"("t Action") -> ()
  n3 = local write "SerialNumber t"("SerialNumber t") -> ()
  n4 = local write "t Motor Settings"("t Motor Settings") -> ()
  n5 = property class="BenchtopStepperControl"(reference="BenchtopStepperControl X", "SerialNumber"="SerialNumber X", "ChannelNumber"=1) -> (reference out=w17:refnum<k24>)  [unwired: 1 in, 1 out]
  n6 = property class="BenchtopStepperControl"(reference="BenchtopStepperControl Y", "SerialNumber"="SerialNumber Y", "ChannelNumber"=2) -> (reference out=w16:refnum<k24>)  [unwired: 1 in, 1 out]
  n7 = property class="KCubeStepperControl"(reference="KCubeStepperControl Z", "SerialNumber"="SerialNumber Z", "ChannelNumber"=3) -> (reference out=w39:refnum<k24>)  [unwired: 1 in, 1 out]
  n8 = invoke class="BenchtopStepperControl" method="CreateDevice"(reference=w17) -> (reference out=w46:refnum<k24>)  [unwired: 2 in, 2 out]
  n9 = invoke class="BenchtopStepperControl" method="CreateDevice"(reference=w16) -> (reference out=w47:refnum<k24>)  [unwired: 2 in, 2 out]
  n10 = invoke class="KCubeStepperControl" method="CreateDevice"(reference=w39) -> (reference out=w38:refnum<k24>)  [unwired: 2 in, 2 out]
  n11 = property class="BenchtopStepperControl"(reference=w46) -> ("BenchtopStepperMotor"=w45:refnum<k24>)  [unwired: 1 in, 2 out]
  n12 = property class="BenchtopStepperControl"(reference=w47) -> ("BenchtopStepperMotor"=w31:refnum<k24>)  [unwired: 1 in, 2 out]
  n13 = property class="KCubeStepperControl"(reference=w38) -> ("Device"=w33:refnum<k24>)  [unwired: 1 in, 2 out]
  n14 = while {
    tunnel: w31 -> [w56]
    tunnel: w45 -> [w60]
    tunnel: [w58] -> w44
    tunnel: [w54] -> w43
    tunnel: [w59] -> w5
    tunnel: [w62] -> w35
    tunnel: [w63] -> w34
    tunnel: w33 -> [w64]
    stop <- w50 stop-if-true
    # "Motor Initialization Loop"
    n15 = flat-sequence {
      tunnel: [w73] -> w49
      tunnel: [w72] -> w48
      frame #0 {
        n16 = local read "KCubeStepperControl t"() -> (w69:refnum<k24>)
        n17 = local read "SerialNumber t"() -> (w68:string)
        n18 = local read "t Motor Settings"() -> (w67:T2)
        n19 = call "ActionEngine(V2).vi"("ChannelNumber"=4, "Settings"=w67, "SerialNumber"=w68, "KCubeStepperControl"=w69, "Action"=ActionEngineEnum."Open Connection") -> ()  [unwired: 4 in, 2 out]
      }
      frame #1 {
        # "I think this is required to go idle"
        n20 = local read "KCubeStepperControl t"() -> (w76:refnum<k24>)
        n21 = local read "SerialNumber t"() -> (w77:string)
        n22 = local read "t Motor Settings"() -> (w78:T2)
        n23 = call "ActionEngine(V2).vi"("ChannelNumber"=4, "Settings"=w78, "SerialNumber"=w77, "KCubeStepperControl"=w76, "Action"=ActionEngineEnum."Done") -> ("error out"=w72:errorcluster, "Current Position"=w73:dbl)  [unwired: 4 in]
      }
    }
    n24 = invoke class="StepperMotorChannel" method="IsSettingsInitialized"(reference=w56) -> (reference out=w54:refnum<k24>, error out=w55:errorcluster, "IsSettingsInitialized"=w53:bool)  [unwired: 2 in]
    n25 = invoke class="StepperMotorChannel" method="IsSettingsInitialized"(reference=w60, error in=w55) -> (reference out=w59:refnum<k24>, error out=w58:errorcluster, "IsSettingsInitialized"=w57:bool)  [unwired: 1 in]
    n26 = invoke class="KCubeStepper" method="IsSettingsInitialized"(reference=w64) -> (reference out=w62:refnum<k24>, error out=w63:errorcluster, "IsSettingsInitialized"=w61:bool)  [unwired: 2 in]
    n27 = local read "Halt program"() -> (w52:bool)
    n28 = And(x=w61, y=w53) -> (x .and. y?=w65:bool)
    n29 = And(x=w57, y=w65) -> (x .and. y?=w51:bool)
    n30 = Wait (ms)(milliseconds to wait=u32 50) -> ()  [unwired: 1 out]
    n31 = Or(x=w51, y=w52) -> (x .or. y?=w50:bool)
    n32 = local write "t - Current Position (mm)"(w49) -> ()
    n33 = local write "t error out"(w48) -> ()
  }
  "X stepper reference" <- w5
  n34 = local write "Halt program"(w11) -> ()
  n35 = local write "Do Linescan"(w11) -> ()
  n36 = local write "Halt linescan"(w11) -> ()
  n37 = while {
    shift-right: [w82] -> _
    shift-left: Control_PRISMRasterScan_ProtocolsLoop."Sit Idle" -> [w79]
    shift-right: [w81] -> _
    shift-left: _ -> [w80]
    stop <- w84 stop-if-true
    w83 = 5
    n38 = case shown="\"Initialize Linescan\"" w79 {
      tunnel: w83 -> [w87 _ _ w135 _ _ _ _]
      tunnel: [w86 Control_PRISMRasterScan_ProtocolsLoop."Update Linescan target" Control_PRISMRasterScan_ProtocolsLoop."Move linescan and wait" w134 Control_PRISMRasterScan_ProtocolsLoop."Sit Idle" Control_PRISMRasterScan_ProtocolsLoop."Sit Idle" Control_PRISMRasterScan_ProtocolsLoop."Sit Idle" Control_PRISMRasterScan_ProtocolsLoop."Sit Idle"] -> w82
      tunnel: [w85 w101 w118 w131 w165 w174 w186 w195] -> w81
      tunnel: w80 -> [w85 _ w118 w131 w165 w174 w186 w195]
      frame "Sit Idle", Default {
        n39 = event shown="[1] \"Generate # points (cursors 1&2)\": Value Change" {
          selector: _ -> [_ _ _ _ _]
          dyn-events: _ -> [_ _ _ _ _]
          timeout: w87 -> [_ _ _ _ _]
          tunnel: [Control_PRISMRasterScan_ProtocolsLoop."Sit Idle" w90 w96 Control_PRISMRasterScan_ProtocolsLoop."Move to stored position" Control_PRISMRasterScan_ProtocolsLoop."Store target position"] -> w86
          event Timeout {
            n40 = event-data() -> ()  [unwired: 1 in, 3 out]
            n41 = local write "Protocol status"("Ready for protocol!") -> ()
          }
          event "Generate\n# points\n(cursors 1&2)": Value Change {
            n42 = event-data() -> ("NewVal"=w93:bool)  [unwired: 1 in]
            n43 = Select(t=Control_PRISMRasterScan_ProtocolsLoop."Generate linescan points", s=w93, f=Control_PRISMRasterScan_ProtocolsLoop."Sit Idle") -> (s? t:f=w90:T6)
          }
          event "Do Linescan": Value Change {
            n44 = event-data() -> ("NewVal"=w97:bool)  [unwired: 1 in]
            n45 = Select(t=Control_PRISMRasterScan_ProtocolsLoop."Initialize Linescan", s=w97, f=Control_PRISMRasterScan_ProtocolsLoop."Sit Idle") -> (s? t:f=w96:T6)
          }
          event "Move to\nstored position": Value Change {
            n46 = event-data() -> ()  [unwired: 1 in, 1 out]
          }
          event "Store target\nposition to": Value Change {
            n47 = event-data() -> ()  [unwired: 1 in, 6 out]
          }
        }
      }
      frame "Initialize Linescan" {
        n48 = flat-sequence {
          tunnel: ["Linescan points\n(relative x,y, microns)"] -> w101
          frame #0 {
            # "# of points in our list"
            n49 = Array Size(array="Linescan points\n(relative x,y, microns)") -> (size(s)=w108:i32[])
            n50 = Index Array(array=w108, index=0) -> (element=w107:i32)
            n51 = call "LineScanCounterAE.vi"("Number of points"=w107, "Accumulate to #"="Linescan Accumulations", "Task"=Control_LineScanCounterAE."Initialize") -> ()  [unwired: 2 in, 7 out]
          }
          frame #1 {
            n52 = control-ref of="Current\naccumulation"() -> (w110:refnum<vi>)
            n53 = control-ref of="Current point"() -> (w109:refnum<vi>)
            n54 = call "LineScanCounterAE.vi"("# Accumulated (reference)"=w110, "Current point index (reference)"=w109, "Task"=Control_LineScanCounterAE."Attach indicators") -> ()  [unwired: 2 in, 7 out]
          }
        }
        n55 = local write "Protocol status"("Initializing linescan...") -> ()
      }
      frame "Update Linescan target" {
        w121 = 1000
        # "Here instead we could compute z based on some xy if we wanted"
        # "Found what point we're on, and index our coordinates there"
        # "Update target"
        n56 = call "LineScanCounterAE.vi"("Task"=Control_LineScanCounterAE."Query" ("Enum")) -> ("Current point index"=w119:i32)  [unwired: 4 in, 6 out]
        n57 = local read "Origin coordinate"() -> (w116:T4)
        n58 = Index Array(array=w118, index (row) #1=w119, index (col) #1=0, index (row) #2=w119, index (col) #2=1) -> (element #1=w130:dbl, element #2=w129:dbl)
        n59 = Unbundle(w116) -> ("X coord (mm)"=w113:dbl, "Y coord (mm)"=w114:dbl, "Z coord (mm)"=w115:dbl, "t coord (mm)"=w112:dbl)
        n60 = Divide(x=w130, y=w121) -> (x/y=w127:dbl)
        n61 = Divide(x=w129, y=w121) -> (x/y=w128:dbl)
        n62 = Add(x=w113, y=w127) -> (x+y=w126:dbl)
        n63 = Subtract(x=w114, y=w128) -> (x-y=w125:dbl)
        n64 = Bundle(w126, w125, "Z coord (mm)"=w115, "t coord (mm)"=w112) -> (w124:T9)  [unwired: 1 in]
        n65 = local write "Target coordinate"(w124) -> ()
      }
      frame "Move linescan and wait" {
        n66 = flat-sequence {
          tunnel: w135 -> [w138]
          tunnel: w135 -> [w147]
          tunnel: [w145] -> w132
          tunnel: [w155] -> w133
          tunnel: w132 -> [w155]
          tunnel: [w163] -> w134
          tunnel: w133 -> [w161]
          frame #0 {
            n67 = property on="Move to target" class="Bool (strict)"("Val(Sgnl)"=TRUE) -> ()  [unwired: 2 in, 2 out]
          }
          frame #1 {
            # "Wait for move to complete"
            n68 = while {
              tunnel: w138 -> [w139]
              stop <- w140 stop-if-true
              n69 = property on="Move to target" class="Bool (strict)"() -> ("Value"=w143:bool)  [unwired: 2 in, 2 out]
              n70 = property on="Halt program" class="Bool (strict)"() -> ("Value"=w141:bool)  [unwired: 2 in, 2 out]
              n71 = Not(x=w143) -> (.not. x?=w142:bool)
              n72 = Or(x=w142, y=w141) -> (x .or. y?=w140:bool)
              n73 = Wait (ms)(milliseconds to wait=w139) -> ()  [unwired: 1 out]
            }
            n74 = local write "Protocol status"("Moving to point...") -> ()
          }
          frame #2 {
            # "Ensure we're activated"
            n75 = call "LineScanCounterAE.vi"("Task"=Control_LineScanCounterAE."Activate") -> ()  [unwired: 4 in, 7 out]
          }
          frame #3 {
            # "Wait till done with point"
            n76 = while {
              tunnel: w147 -> [w153]
              tunnel: [w148] -> w145
              stop <- w151 stop-if-true
              n77 = local read "Halt linescan"() -> (w148:bool)
              n78 = local read "Halt program"() -> (w152:bool)
              n79 = call "LineScanCounterAE.vi"("Task"=Control_LineScanCounterAE."Query") -> ("Done with point"=w149:bool)  [unwired: 4 in, 6 out]
              n80 = Wait (ms)(milliseconds to wait=w153) -> ()  [unwired: 1 out]
              n81 = Or(x=w152, y=w148) -> (x .or. y?=w150:bool)
              n82 = Or(x=w149, y=w150) -> (x .or. y?=w151:bool)
            }
            n83 = local write "Protocol status"("Waiting for data collection...") -> ()
          }
          frame #4 {
            # "Done with that\npoint, tell counter\nwe're ready to move on"
            n84 = call "LineScanCounterAE.vi"("Task"=Control_LineScanCounterAE."Increment Point") -> ()  [unwired: 4 in, 7 out]
          }
          frame #5 {
            # "If we are done,\ncounter inactivates\nfor us automatically"
            n85 = call "LineScanCounterAE.vi"("Task"=Control_LineScanCounterAE."Query") -> ("Active"=w159:bool)  [unwired: 4 in, 6 out]
            n86 = Not(x=w159) -> (.not. x?=w160:bool)
            n87 = Or(x=w160, y=w161) -> (x .or. y?=w162:bool)
            n88 = Select(t=Control_PRISMRasterScan_ProtocolsLoop."Finalize linescan", s=w162, f=Control_PRISMRasterScan_ProtocolsLoop."Update Linescan target") -> (s? t:f=w163:T6)
          }
        }
      }
      frame "Finalize linescan" {
        # "In case we arrived here by some error, close out the linescan"
        # "Here we can return to origin"
        n89 = flat-sequence {
          frame #0 {
            n90 = property on="Move to origin" class="Bool (strict)"("Val(Sgnl)"=FALSE) -> ()  [unwired: 2 in, 2 out]
            n91 = call "LineScanCounterAE.vi"("Task"=Control_LineScanCounterAE."Deactivate" ("Enum")) -> ()  [unwired: 4 in, 7 out]
          }
          frame #1 {
            n92 = local write "Do Linescan"(FALSE) -> ()
          }
          frame #2 {
            n93 = Wait (ms)(milliseconds to wait=500) -> ()  [unwired: 1 out]
            n94 = local write "Halt linescan"(FALSE) -> ()
            n95 = local write "Protocol status"("Linescan complete!") -> ()
          }
        }
      }
      frame "Move to stored position" {
        n96 = flat-sequence {
          tunnel: [w177] -> w173
          tunnel: w173 -> [w183]
          frame #0 {
            n97 = local read "Stored positions"() -> (w176:T5)
            n98 = Search 1D Array(1D array="Move to\nstored position", element=TRUE) -> (index of element=w177:i32)  [unwired: 1 in]
            n99 = Index Array(array=w176, index=w177) -> (element=w178:T4)
            n100 = local write "Target coordinate"(w178) -> ()
          }
          frame #1 {
            n101 = Format Into String(w183) -> (resulting string=w182:string)  [unwired: 3 in, 1 out]
            n102 = Concatenate Strings("Moving to coordinates ", w182) -> (w181:string)
            n103 = local write "Protocol status"(w181) -> ()
          }
          frame #2 {
            n104 = property on="Move to target" class="Bool (strict)"("Val(Sgnl)"=TRUE) -> ()  [unwired: 2 in, 2 out]
          }
          frame #3 {
            n105 = invoke on="Move to\nstored position" class="Arr (strict)" method="Reinit To Default"() -> ()  [unwired: 3 in, 3 out]
          }
        }
      }
      frame "Store target position" {
        n106 = flat-sequence {
          frame #0 {
            n107 = local read "Target coordinate"() -> (w189:T4)
            n108 = local read "Stored positions"() -> (w188:T5)
            n109 = Search 1D Array(1D array="Store target\nposition to", element=TRUE) -> (index of element=w191:i32)  [unwired: 1 in]
            n110 = Replace Array Subset(array=w188, new element=w189, index=w191) -> (w190:T5)
            n111 = local write "Stored positions"(w190) -> ()
          }
          frame #1 {
            n112 = Wait (ms)(milliseconds to wait=500) -> ()  [unwired: 1 out]
          }
          frame #2 {
            n113 = invoke on="Store target\nposition to" class="Arr (strict)" method="Reinit To Default"() -> ()  [unwired: 3 in, 3 out]
          }
        }
      }
      frame "Generate linescan points" {
        # "Ultimately we'll next go \nto \"plot linescan points\""
        n114 = flat-sequence {
          frame #0 {
            # "Minimum of 2"
            # "dy"
            # "dx"
            # "Make # points the row (1st) dimension"
            # "All y points"
            # "All x points"
            n115 = property on="Amplitude" class="IntGraph (strict)"() -> ("CrsrLis"=w215:T10)  [unwired: 2 in, 2 out]
            n116 = Index Array(array=w215, index #1=1, index #2=0) -> (element #1=w211:T11, element #2=w212:T11)
            n117 = Unbundle By Name(w211) -> ("Position.X"=w210:dbl, "Position.Y"=w209:dbl)
            n118 = Unbundle By Name(w212) -> ("Position.X"=w205:dbl, "Position.Y"=w206:dbl)
            n119 = Decrement(x="# Points") -> (x-1=w197:i32)
            n120 = Subtract(x=w210, y=w205) -> (x-y=w208:dbl)
            n121 = Subtract(x=w209, y=w206) -> (x-y=w207:dbl)
            n122 = Divide(x=w208, y=w197) -> (x/y=w203:dbl)
            n123 = Divide(x=w207, y=w197) -> (x/y=w204:dbl)
            n124 = for {
              N: "# Points" -> [_]
              tunnel: w206 -> [w219]
              tunnel: w205 -> [w220]
              tunnel: w204 -> [w224]
              tunnel: w203 -> [w222]
              tunnel: [w217] -> w202 mode=indexing
              tunnel: [w216] -> w201 mode=indexing
              i -> [w223]
              # "x0"
              # "y0"
              n125 = Multiply(x=w222, y=w223) -> (x*y=w221:dbl)
              n126 = Multiply(x=w223, y=w224) -> (x*y=w218:dbl)
              n127 = Add(x=w221, y=w220) -> (x+y=w217:dbl)
              n128 = Add(x=w218, y=w219) -> (x+y=w216:dbl)
            }
            n129 = Build Array(w202, w201) -> (w199:dbl[][])
            n130 = Transpose 2D Array(2D array=w199) -> (transposed array=w200:dbl[][])
            n131 = local write "Linescan points\n(relative x,y, microns)"(w200) -> ()
          }
          frame #1 {
            n132 = property on="Generate\n# points\n(cursors 1&2)" class="Bool (strict)"("Value"=FALSE) -> ()  [unwired: 2 in, 2 out]
          }
        }
      }
    }
    n133 = Wait (ms)(milliseconds to wait=w83) -> ()  [unwired: 1 out]
    n134 = property on="Halt program" class="Bool (strict)"() -> ("Value"=w84:bool)  [unwired: 2 in, 2 out]
  }
  n135 = property on="Y stepper reference" class="Ref (strict)" props=["Value"]() -> ()  [unwired: 2 in, 3 out]
  n136 = property on="X stepper reference" class="Ref (strict)" props=["Value"]() -> ()  [unwired: 2 in, 3 out]
  n137 = invoke class="StepperMotorChannel" method="EnableDevice"(reference=w43, error in=w44) -> (reference out=w12:refnum<k24>, error out=w42:errorcluster)  [unwired: 1 in, 1 out]
  "Y stepper reference" <- w12
  n138 = invoke class="KCubeStepper" method="EnableDevice"(reference=w35, error in=w34) -> (reference out=w9:refnum<k24>)  [unwired: 1 in, 2 out]
  n139 = while {
    shift-right: [w231] -> _
    shift-left: Control_PRISMRasterScan_ActivityLoop."Sit Idle" -> [w232]
    tunnel: w12 -> [w227]
    tunnel: w5 -> [w226]
    tunnel: w9 -> [w228]
    tunnel: [w228] -> w8
    tunnel: [w227] -> w7
    tunnel: [w226] -> w6
    stop <- w230 stop-if-true
    w229 = 5
    n140 = case shown="\"Update origin or target position\"" w232 {
      tunnel: [w234 w266 Control_PRISMRasterScan_ActivityLoop."Sit Idle" Control_PRISMRasterScan_ActivityLoop."Sit Idle"] -> w231
      tunnel: w229 -> [w233 _ _ _]
      tunnel: w227 -> [_ w265 w286 _]
      tunnel: w226 -> [_ w264 w285 _]
      tunnel: w228 -> [_ w263 w287 _]
      frame "Sit Idle", Default {
        n141 = event shown="[1] \"Amplitude\": Cursor Release" {
          selector: _ -> [_ _ _ _ _]
          dyn-events: _ -> [_ _ _ _ _]
          timeout: w233 -> [_ _ _ _ _]
          tunnel: [Control_PRISMRasterScan_ActivityLoop."Sit Idle" _ w251 w255 w259] -> w234
          event Timeout {
            n142 = event-data() -> ()  [unwired: 1 in, 3 out]
          }
          event "Amplitude": Cursor Release {
            w244 = 1000
            # "Update the target coordinate based on cursor position in amplitude intensity plot"
            n143 = event-data() -> ("CursLoc"=w250:cluster{"X":dbl, "Y":dbl})  [unwired: 1 in, 3 out]
            n144 = Unbundle(w250) -> ("X"=w243:dbl, "Y"=w242:dbl)
            n145 = property on="Origin coordinate" class="Clust (strict)"() -> ("Value"=w239:T4)  [unwired: 2 in, 2 out]
            n146 = local read "Target coordinate"() -> (w241:T4)
            n147 = Divide(x=w243, y=w244) -> (x/y=w249:dbl)
            n148 = Divide(x=w242, y=w244) -> (x/y=w248:dbl)
            n149 = Unbundle(w239) -> ("X coord (mm)"=w238:dbl, "Y coord (mm)"=w237:dbl)  [unwired: 2 out]
            n150 = Add(x=w238, y=w249) -> (x+y=w246:dbl)
            n151 = Subtract(x=w237, y=w248) -> (x-y=w247:dbl)
            n152 = Unbundle(w241) -> ("Z coord (mm)"=w240:dbl, "t coord (mm)"=w236:dbl)  [unwired: 2 out]
            n153 = Bundle(w246, w247, "Z coord (mm)"=w240, "t coord (mm)"=w236) -> (w245:T9)  [unwired: 1 in]
            n154 = local write "Target coordinate"(w245) -> ()
          }
          event "Move to origin": Value Change {
            n155 = event-data() -> ("NewVal"=w254:bool)  [unwired: 1 in]
            n156 = Select(t=Control_PRISMRasterScan_ActivityLoop."Move to origin", s=w254, f=Control_PRISMRasterScan_ActivityLoop."Sit Idle") -> (s? t:f=w251:T7)
          }
          event "Move to target": Value Change {
            n157 = event-data() -> ("NewVal"=w258:bool)  [unwired: 1 in]
            n158 = Select(t=Control_PRISMRasterScan_ActivityLoop."Move to target", s=w258, f=Control_PRISMRasterScan_ActivityLoop."Sit Idle") -> (s? t:f=w255:T7)
          }
          event "Update origin", "Update target": Value Change {
            n159 = event-data() -> ("NewVal"=w262:bool)  [unwired: 1 in]
            n160 = Select(t=Control_PRISMRasterScan_ActivityLoop."Update origin or target position", s=w262, f=Control_PRISMRasterScan_ActivityLoop."Sit Idle") -> (s? t:f=w259:T7)
          }
        }
      }
      frame "Move to target" {
        n161 = flat-sequence {
          tunnel: w265 -> [w274]
          tunnel: w264 -> [w273]
          tunnel: w263 -> [w270]
          tunnel: [Control_PRISMRasterScan_ActivityLoop."Sit Idle"] -> w266
          frame #0 {
            w267 = 0
            n162 = local read "Target coordinate"() -> (w272:T4)
            n163 = Unbundle(w272) -> ("X coord (mm)"=w277:dbl, "Y coord (mm)"=w276:dbl, "Z coord (mm)"=w271:dbl)  [unwired: 1 out]
            n164 = invoke class="StepperMotorChannel" method="SetMoveAbsolutePosition"(reference=w273, "position"=w277) -> (reference out=w275:refnum<k24>, error out=w278:errorcluster)  [unwired: 2 in, 2 out]
            n165 = invoke class="StepperMotorChannel" method="SetMoveAbsolutePosition"(reference=w274, "position"=w276) -> (reference out=w280:refnum<k24>, error out=w279:errorcluster)  [unwired: 2 in, 2 out]
            n166 = invoke class="KCubeStepper" method="SetMoveAbsolutePosition"(reference=w270, "position"=w271) -> (reference out=w269:refnum<k24>, error out=w268:errorcluster)  [unwired: 2 in, 2 out]
            n167 = invoke class="StepperMotorChannel" method="MoveAbsolute"(reference=w275, error in=w278, "waitTimeout"=w267) -> ()  [unwired: 1 in, 4 out]
            n168 = invoke class="StepperMotorChannel" method="MoveAbsolute"(reference=w280, error in=w279, "waitTimeout"=w267) -> ()  [unwired: 1 in, 4 out]
            n169 = invoke class="KCubeStepper" method="MoveAbsolute"(reference=w269, error in=w268, "waitTimeout"=w267) -> ()  [unwired: 1 in, 4 out]
          }
          frame #1 {
            n170 = local read "Settle Time Y"() -> (w281:u32)
            n171 = Wait (ms)(milliseconds to wait=w281) -> ()  [unwired: 1 out]
          }
          frame #2 {
            n172 = local write "Move to target"(FALSE) -> ()
          }
        }
      }
      frame "Update origin or target position" {
        n173 = flat-sequence {
          tunnel: w287 -> [w294]
          tunnel: w286 -> [w295]
          tunnel: w285 -> [w296]
          frame #0 {
            w303 = 409600
            # "Position as # microscops"
            # "Microsteps per mm"
            n174 = invoke class="StepperMotorChannel" method="GetPositionCounter"(reference=w295) -> ("GetPositionCounter"=w301:i32)  [unwired: 2 in, 2 out]
            n175 = invoke class="StepperMotorChannel" method="GetPositionCounter"(reference=w296) -> ("GetPositionCounter"=w302:i32)  [unwired: 2 in, 2 out]
            n176 = flat-sequence {
              tunnel: [w304] -> w289
              tunnel: w289 -> [w315]
              tunnel: [w315] -> w288
              frame #0 {
                n177 = local read "KCubeStepperControl t"() -> (w307:refnum<k24>)
                n178 = local read "SerialNumber t"() -> (w308:string)
                n179 = local read "t Motor Settings"() -> (w309:T2)
                n180 = call "ActionEngine(V2).vi"("ChannelNumber"=4, "Settings"=w309, "SerialNumber"=w308, "KCubeStepperControl"=w307, "Action"=ActionEngineEnum."Get Position") -> ("Current Position"=w304:dbl)  [unwired: 4 in, 1 out]
              }
              frame #1 {
                n181 = local read "KCubeStepperControl t"() -> (w312:refnum<k24>)
                n182 = local read "SerialNumber t"() -> (w311:string)
                n183 = local read "t Motor Settings"() -> (w310:T2)
                n184 = call "ActionEngine(V2).vi"("ChannelNumber"=4, "Settings"=w310, "SerialNumber"=w311, "KCubeStepperControl"=w312, "Action"=ActionEngineEnum."Done") -> ()  [unwired: 4 in, 2 out]
              }
            }
            n185 = invoke class="KCubeStepper" method="GetPositionCounter"(reference=w294) -> ("GetPositionCounter"=w297:i32)  [unwired: 2 in, 2 out]
            n186 = Divide(x=w297, y=2184560.64) -> (x/y=w298:dbl)
            n187 = Divide(x=w302, y=w303) -> (x/y=w300:dbl)
            n188 = Divide(x=w301, y=w303) -> (x/y=w299:dbl)
            n189 = local read "Update target"() -> (w291:bool)
            n190 = local read "Update origin"() -> (w292:bool)
            n191 = Bundle(w300, w299, w298, "Current Position"=w288) -> (w290:cluster{dbl, dbl, dbl, "Current Position":dbl})  [unwired: 1 in]
            n192 = case shown="True" w291 {
              tunnel: w290 -> [_ w316]
              frame False {
              }
              frame True {
                n193 = local write "Target coordinate"(w316) -> ()
              }
            }
            n194 = case shown="True" w292 {
              tunnel: w290 -> [_ w317]
              frame False {
              }
              frame True {
                n195 = local write "Origin coordinate"(w317) -> ()
              }
            }
          }
          frame #1 {
            w318 = FALSE
            n196 = local write "Update origin"(w318) -> ()
            n197 = local write "Update target"(w318) -> ()
          }
        }
      }
      frame "Move to origin" {
        n198 = flat-sequence {
          frame #0 {
            n199 = local read "Origin coordinate"() -> (w320:T4)
            n200 = local write "Target coordinate"(w320) -> ()
          }
          frame #1 {
            n201 = property on="Move to target" class="Bool (strict)"("Val(Sgnl)"=TRUE) -> ()  [unwired: 2 in, 2 out]
            n202 = local write "Move to origin"(FALSE) -> ()
          }
        }
      }
    }
    n203 = Wait (ms)(milliseconds to wait=w229) -> ()  [unwired: 1 out]
    n204 = property on="Halt program" class="Bool (strict)"() -> ("Value"=w230:bool)  [unwired: 2 in, 2 out]
  }
  n205 = invoke class="StepperMotorChannel" method="EnableDevice"(reference=w5, error in=w42) -> (reference out=w41:refnum<k24>, error out=w32:errorcluster)  [unwired: 1 in, 1 out]
  n206 = Open Python Session(python version="3.9", python path=path "C:/Users/mnopl/anaconda3/python.exe") -> (session out=w28:refnum<k35>, error out=w26:errorcluster)  [unwired: 1 in]
  n207 = invoke class="StepperMotorChannel" method="Disconnect"(reference=w6) -> ()  [unwired: 2 in, 3 out]
  n208 = invoke class="StepperMotorChannel" method="Disconnect"(reference=w7) -> ()  [unwired: 2 in, 3 out]
  n209 = invoke class="KCubeStepper" method="Disconnect"(reference=w8) -> ()  [unwired: 2 in, 3 out]
  n210 = while {
    tunnel: w12 -> [w325]
    tunnel: w41 -> [w326]
    tunnel: w32 -> [w335]
    tunnel: w28 -> [w334]
    tunnel: path "C:/Users/mnopl/Desktop/Software/mnOPSuite/PRISM/python/prism_scanning.py" -> [w333]
    tunnel: w26 -> [w332]
    tunnel: [w331] -> w25
    tunnel: [w330] -> w24
    tunnel: [w329] -> w23
    tunnel: [w328] -> w22
    stop <- w323 stop-if-true
    # "Start scan"
    n211 = Wait (ms)(milliseconds to wait=50) -> ()  [unwired: 1 out]
    n212 = case shown="True" "Save Image" {
      frame False {
      }
      frame True {
        n213 = flat-sequence {
          tunnel: [w340] -> w339
          tunnel: w339 -> [w355]
          tunnel: [w355] -> w338
          tunnel: w338 -> [w368]
          frame #0 {
            w348 = "%g"
            n214 = Path To String(path="Path to save image") -> (string=w340:string)
            n215 = Search and Replace String(input string=w340, search string="(.txt)$", replace string="_phase.txt") -> (result string=w353:string)  [unwired: 5 in, 3 out]
            n216 = Search and Replace String(input string=w340, search string="(.txt)*$", replace string="_amplitude.txt") -> (result string=w341:string)  [unwired: 5 in, 3 out]
            n217 = property on="Phase" class="IntGraph (strict)"() -> ("Value"=w343:dbl[][])  [unwired: 2 in, 2 out]
            n218 = property on="Amplitude" class="IntGraph (strict)"() -> ("Value"=w342:dbl[][])  [unwired: 2 in, 2 out]
            n219 = Array To Spreadsheet String(array=w343, 3:w348) -> (spreadsheet string=w354:string)  [unwired: 1 in]
            n220 = Array To Spreadsheet String(array=w342, 3:w348) -> (spreadsheet string=w349:string)  [unwired: 1 in]
            n221 = String To Path(string=w353) -> (path=w352:path)
            n222 = String To Path(string=w341) -> (path=w351:path)
            n223 = Write to Text File(file (use dialog)=w352, text=w354) -> ()  [unwired: 2 in, 3 out]
            n224 = Write to Text File(file (use dialog)=w351, text=w349) -> ()  [unwired: 2 in, 3 out]
          }
          frame #1 {
            n225 = invoke on="Amplitude" class="IntGraph (strict)" method="Get Image"() -> ("image data"=w361:T12)  [unwired: 6 in, 5 out]
            n226 = Search and Replace String(input string=w355, search string="(.txt)$", replace string="_amplitude.png") -> (result string=w363:string)  [unwired: 5 in, 3 out]
            n227 = String To Path(string=w363) -> (path=w362:path)
            n228 = call <vilib>:"Write PNG File.vi"("image data"=w361, "path to PNG file"=w362) -> ()  [unwired: 8 in, 2 out]
            n229 = invoke on="Phase" class="IntGraph (strict)" method="Get Image"() -> ("image data"=w357:T12)  [unwired: 6 in, 5 out]
            n230 = Search and Replace String(input string=w355, search string="(.txt)$", replace string="_phase.png") -> (result string=w358:string)  [unwired: 5 in, 3 out]
            n231 = String To Path(string=w358) -> (path=w356:path)
            n232 = call <vilib>:"Write PNG File.vi"("image data"=w357, "path to PNG file"=w356) -> ()  [unwired: 8 in, 2 out]
          }
          frame #2 {
            n233 = local write "Save Image"(FALSE) -> ()
            n234 = Concatenate Strings("Image successfully saved to:" ("message"), "\r", w368) -> (w369:string)
            n235 = One Button Dialog(message=w369, button name ("OK")="OK") -> ()  [unwired: 1 out]
          }
        }
      }
    }
    n236 = case shown="True" "Move to cursor 1" {
      tunnel: w326 -> [_ w385]
      tunnel: w325 -> [_ w381]
      frame False {
      }
      frame True {
        w379 = 1000
        # "This is a cludge:  The scan is actually incrementing y DOWN with increasing step, inverting the motor"
        # "This takes the coordinate of last cursor"
        n237 = property on="Amplitude" class="IntGraph (strict)"() -> ("CrsrLis"=w390:T10)  [unwired: 2 in, 2 out]
        n238 = for {
          tunnel: w390 -> [w393] mode=indexing
          tunnel: [w392] -> w378
          tunnel: [w391] -> w380
          n239 = Unbundle By Name(w393) -> ("Position.X"=w392:dbl, "Position.Y"=w391:dbl)
        }
        n240 = property on="Origin coordinate" class="Clust (strict)"() -> ("Value"=w374:T4)  [unwired: 2 in, 2 out]
        n241 = Divide(x=w378, y=w379) -> (x/y=w377:dbl)
        n242 = Divide(x=w380, y=w379) -> (x/y=w375:dbl)
        n243 = Unbundle(w374) -> ("X coord (mm)"=w373:dbl, "Y coord (mm)"=w372:dbl)  [unwired: 2 out]
        n244 = Add(x=w373, y=w377) -> (x+y=w386:dbl)
        n245 = Subtract(x=w372, y=w375) -> (x-y=w376:dbl)
        n246 = invoke class="StepperMotorChannel" method="SetMoveAbsolutePosition"(reference=w385, "position"=w386) -> (reference out=w389:refnum<k24>, error out=w388:errorcluster)  [unwired: 2 in, 2 out]
        n247 = invoke class="StepperMotorChannel" method="SetMoveAbsolutePosition"(reference=w381, "position"=w376) -> (reference out=w384:refnum<k24>, error out=w383:errorcluster)  [unwired: 2 in, 2 out]
        n248 = invoke class="StepperMotorChannel" method="MoveAbsolute"(reference=w389, error in=w388, "waitTimeout"=0) -> ()  [unwired: 1 in, 4 out]
        n249 = invoke class="StepperMotorChannel" method="MoveAbsolute"(reference=w384, error in=w383, "waitTimeout"=0) -> ()  [unwired: 1 in, 4 out]
      }
    }
    n250 = case shown="True" "?" {
      tunnel: w326 -> [w395 w402]
      tunnel: w325 -> [_ w401]
      tunnel: w335 -> [w394 w400]
      tunnel: w334 -> [w397 w409]
      tunnel: w333 -> [_ w408]
      tunnel: w332 -> [w396 w407]
      tunnel: [w397 w406] -> w331
      tunnel: [w396 w405] -> w330
      tunnel: [w395 w404] -> w329
      tunnel: [w394 w403] -> w328
      frame False {
      }
      frame True {
        # "Scan sequence: Loops, wait, return to origin, done"
        n251 = flat-sequence {
          tunnel: [w413] -> w399
          tunnel: [w412] -> w398
          frame #0 {
            n252 = property on="Update origin" class="Bool (strict)"("Val(Sgnl)"=TRUE) -> ()  [unwired: 2 in, 2 out]
          }
          frame #1 {
            n253 = while {
              stop <- w411 continue-if-true
              n254 = local read "Update origin"() -> (w411:bool)
            }
          }
          frame #2 {
            n255 = property on="Origin coordinate" class="Clust (strict)"() -> ("Value"=w414:T4)  [unwired: 2 in, 2 out]
            n256 = Unbundle(w414) -> ("X coord (mm)"=w413:dbl, "Y coord (mm)"=w412:dbl)  [unwired: 2 out]
          }
        }
        n257 = stacked-sequence {
          tunnel: w401 -> [_ w429 _ w626 _]
          tunnel: w398 -> [_ w426 _ w624 _]
          tunnel: w402 -> [_ w430 _ w625 _]
          tunnel: w400 -> [_ w431 _ _ _]
          tunnel: w399 -> [_ w425 _ w623 _]
          tunnel: w409 -> [_ w436 _ _ _]
          tunnel: w408 -> [_ w435 _ _ _]
          tunnel: w407 -> [_ w434 _ _ _]
          tunnel: [_ w433 _ _ _] -> w406
          tunnel: [_ w432 _ _ _] -> w405
          tunnel: [_ w428 _ _ _] -> w404
          tunnel: [_ w427 _ _ _] -> w403
          frame #0 {
            n258 = local read "Num Of Steps X"() -> (w423:i32)
            n259 = local read "Num Of Steps Y"() -> (w420:i32)
            n260 = local read "Step Size X (um)"() -> (w418:sgl)
            n261 = local read "Step Size Y (um)"() -> (w416:sgl)
            n262 = Divide(x=w420, y=-2) -> (x/y=w421:dbl)
            n263 = Divide(x=w423, y=-2) -> (x/y=w424:dbl)
            n264 = property on="Amplitude" class="IntGraph (strict)"("XScale.Multiplier"=w418) -> ()  [unwired: 2 in, 2 out]
            n265 = property on="Amplitude" class="IntGraph (strict)"("YScale.Multiplier"=w416) -> ()  [unwired: 2 in, 2 out]
            n266 = Multiply(x=w416, y=w421) -> (x*y=w415:dbl)
            n267 = Multiply(x=w418, y=w424) -> (x*y=w417:dbl)
            n268 = property on="Amplitude" class="IntGraph (strict)"("XScale.Offset"=w417) -> ()  [unwired: 2 in, 2 out]
            n269 = property on="Amplitude" class="IntGraph (strict)"("YScale.Offset"=w415) -> ()  [unwired: 2 in, 2 out]
          }
          frame #1 {
            w438 = 0.0
            # "Outer loop: Y-stepper"
            n270 = local read "Num Of Steps X"() -> (w440:i32)
            n271 = local read "Num Of Steps Y"() -> (w441:i32)
            n272 = Re/Im To Complex(1:w438, 2:w438) -> (0:w437:cdb)
            n273 = Initialize Array(w437, w440, w441) -> (w439:cdb[][])
            n274 = while {
              shift-right: [w456] -> _
              shift-left: w439 -> [w457]
              tunnel: [w455] -> w428
              tunnel: w436 -> [w448]
              tunnel: w435 -> [w443]
              tunnel: w434 -> [w454]
              tunnel: [w453] -> w433
              tunnel: [w452] -> w432
              tunnel: w431 -> [w450]
              tunnel: w430 -> [w447]
              tunnel: w429 -> [w446]
              tunnel: w426 -> [w445]
              tunnel: w425 -> [w444]
              tunnel: [w442] -> w427
              i -> [w449]
              stop <- w458 stop-if-true
              # "Y-sequence: Move y, settle y, X-loop"
              n275 = stacked-sequence {
                tunnel: w457 -> [_ w485]
                tunnel: w454 -> [_ w484]
                tunnel: [_ w492] -> w459
                tunnel: [_ w491] -> w456
                tunnel: [_ w490] -> w455
                tunnel: [_ w489] -> w453
                tunnel: [_ w488] -> w452
                tunnel: [w469 _] -> w451
                tunnel: w450 -> [w465 w487]
                tunnel: w449 -> [w460 w486]
                tunnel: w448 -> [_ w483]
                tunnel: w447 -> [_ w482]
                tunnel: w446 -> [w466 _]
                tunnel: w445 -> [w464 _]
                tunnel: w444 -> [_ w481]
                tunnel: w443 -> [_ w480]
                tunnel: [_ w479] -> w442
                frame #0 {
                  n276 = local read "Step Size Y (um)"() -> (w468:sgl)
                  n277 = local read "Num Of Steps Y"() -> (w474:i32)
                  n278 = Equal?(x=w460, y=w474) -> (x = y?=w472:bool)
                  n279 = Divide(x=w474, y=2) -> (x/y=w461:dbl)
                  n280 = Divide(x=w468, y=1000) -> (x/y=w478:sgl)
                  n281 = local read "Halt program"() -> (w473:bool)
                  n282 = Subtract(x=w461, y=w460) -> (x-y=w476:dbl)
                  n283 = Or(x=w473, y=w472) -> (x .or. y?=w469:bool)
                  n284 = Multiply(x=w478, y=w476) -> (x*y=w477:dbl)
                  n285 = Add(x=w464, y=w477) -> (x+y=w462:dbl)
                  n286 = invoke class="StepperMotorChannel" method="SetMoveAbsolutePosition"(reference=w466, error in=w465, "position"=w462) -> (reference out=w467:refnum<k24>, error out=w475:errorcluster)  [unwired: 1 in, 2 out]
                  n287 = invoke class="StepperMotorChannel" method="MoveAbsolute"(reference=w467, error in=w475, "waitTimeout"=20000) -> ()  [unwired: 1 in, 4 out]
                }
                frame #1 {
                  # "Inner loop: X-stepper"
                  n288 = while {
                    tunnel: w483 -> [w508]
                    tunnel: [w507] -> w490
                    tunnel: [w504] -> w492
                    tunnel: w486 -> [w497]
                    shift-right: [w502] -> w491
                    shift-left: w485 -> [w503]
                    tunnel: w484 -> [w501]
                    tunnel: [w500] -> w489
                    tunnel: [w499] -> w488
                    tunnel: w487 -> [w498]
                    tunnel: w482 -> [w496]
                    tunnel: w481 -> [w495]
                    tunnel: w480 -> [w494]
                    tunnel: [w493] -> w479
                    i -> [w506]
                    stop <- w505 stop-if-true
                    # "X-sequence: Move X, settle X, DAQ & plot"
                    n289 = stacked-sequence {
                      tunnel: w508 -> [_ _ w542]
                      tunnel: [w530 _ _] -> w507
                      tunnel: w498 -> [w529 _ _]
                      tunnel: w506 -> [w521 w533 w540]
                      tunnel: [w523 _ _] -> w505
                      tunnel: ["?" _ _] -> w504
                      tunnel: w503 -> [_ _ w547]
                      tunnel: [_ _ w545] -> w502
                      tunnel: w501 -> [_ _ w546]
                      tunnel: [_ _ w544] -> w500
                      tunnel: [_ _ w543] -> w499
                      tunnel: w497 -> [_ _ w539]
                      tunnel: w496 -> [w512 _ _]
                      tunnel: w495 -> [w511 _ _]
                      tunnel: w494 -> [_ _ w541]
                      tunnel: [w509 _ _] -> w493
                      frame #0 {
                        n290 = local read "Step Size X (um)"() -> (w513:sgl)
                        n291 = local read "Num Of Steps X"() -> (w519:i32)
                        n292 = Equal?(x=w521, y=w519) -> (x = y?=w526:bool)
                        n293 = Divide(x=w519, y=2) -> (x/y=w517:dbl)
                        n294 = Divide(x=w513, y=1000) -> (x/y=w514:sgl)
                        n295 = Subtract(x=w521, y=w517) -> (x-y=w520:dbl)
                        n296 = local read "Halt program"() -> (w525:bool)
                        n297 = Or(x=w525, y=w526) -> (x .or. y?=w524:bool)
                        n298 = Multiply(x=w514, y=w520) -> (x*y=w516:dbl)
                        n299 = Add(x=w511, y=w516) -> (x+y=w527:dbl)
                        n300 = invoke class="StepperMotorChannel" method="SetMoveAbsolutePosition"(reference=w512, error in=w529, "position"=w527) -> (reference out=w531:refnum<k24>, error out=w528:errorcluster)  [unwired: 1 in, 2 out]
                        n301 = invoke class="StepperMotorChannel" method="MoveAbsolute"(reference=w531, error in=w528, "waitTimeout"=0) -> (reference out=w530:refnum<k24>, error out=w509:errorcluster)  [unwired: 1 in, 2 out]
                        n302 = Or(x=w524, y="?") -> (x .or. y?=w523:bool)
                      }
                      frame #1 {
                        # "If i=0, it means we've likely just moved back to start of line, and we should wait a moment"
                        n303 = Equal?(x=0, y=w533) -> (x = y?=w534:bool)
                        n304 = case shown="True" w534 {
                          frame False {
                            n305 = Wait (ms)(milliseconds to wait="Settle Time X") -> ()  [unwired: 1 out]
                          }
                          frame True {
                            n306 = Wait (ms)(milliseconds to wait="Settle Time Y") -> ()  [unwired: 1 out]
                          }
                        }
                      }
                      frame #2 {
                        n307 = case shown="True" "Acquire" {
                          tunnel: w547 -> [w548 w578]
                          tunnel: w546 -> [w549 w574]
                          tunnel: [w548 w571] -> w545
                          tunnel: [w550 w567] -> w544
                          tunnel: [w549 w566] -> w543
                          tunnel: w542 -> [w550 w565]
                          tunnel: w541 -> [_ w564]
                          tunnel: w540 -> [_ w559]
                          tunnel: w539 -> [_ w558]
                          tunnel: "Integration time (s)" -> [w553 w556]
                          frame False {
                            n308 = Multiply(x=w553, y=1000) -> (x*y=w551:dbl)
                            n309 = Wait (ms)(milliseconds to wait=w551) -> ()  [unwired: 1 out]
                          }
                          frame True {
                            w586 = 200000
                            n310 = Multiply(x=w586, y=w556) -> (x*y=w585:dbl)
                            n311 = call "DAQ Assistant"("rate"=w586, "number of samples"=w585) -> ("data"=w584:dynamicdata)  [unwired: 15 in, 2 out]
                            n312 = call "Convert from Dynamic Data"("Dynamic Data Type"=w584) -> ("Array"=w583:dbl[][])  [unwired: 3 in]
                            n313 = Index Array(array=w583, index (row)=0) -> (element=w580:dbl[])  [unwired: 1 in]
                            n314 = Index Array(array=w583, index (row)=1) -> (element=w579:dbl[])  [unwired: 1 in]
                            n315 = call-poly <vilib>:"Mean.vi"("X"=w580) -> ("mean"=w575:dbl)  [unwired: 1 out]
                            n316 = call-poly <vilib>:"Mean.vi"("X"=w579) -> ("mean"=w563:dbl)  [unwired: 1 out]
                            n317 = Subtract(x=w575, y="1st sideband offset") -> (x-y=w557:dbl)
                            n318 = Multiply(x=w563, y="2nd sideband factor") -> (x*y=w562:dbl)
                            n319 = Re/Im To Complex(1:w562, 2:w557) -> (0:w560:cdb)
                            n320 = Replace Array Subset(array=w578, new element=w560, index (row)=w559, index (col)=w558) -> (w571:cdb[][])
                            n321 = Not(x="Auto-level phase") -> (.not. x?=w554:bool)
                            n322 = Complex To Polar(r * e^(i*theta)=w571) -> (r=→"Amplitude":dbl[][], theta=w573:dbl[][])
                            n323 = case shown="False" w554 {
                              tunnel: w574 -> [w608 w620]
                              tunnel: w573 -> [w607 w619]
                              tunnel: [w603 w618] -> w572
                              tunnel: "Phase offset" -> [w604 w617]
                              tunnel: "Px" -> [w606 w616]
                              tunnel: "Py" -> [w605 w615]
                              tunnel: [w601 w614] -> w567
                              tunnel: [w599 w613] -> w566
                              tunnel: w565 -> [w610 w612]
                              tunnel: w564 -> [w598 w611]
                              frame False {
                                n324 = node(w610, w598, "auto_phase_level", w608, w607, w607, w606, w605, w604) -> (w602:refnum<k35>, w600:errorcluster, w603:dbl[][])  [unwired: 4 in, 2 out]
                                n325 = Initialize Array(0.0, 3) -> (w587:dbl[])
                                n326 = node(w602, w598, "get_level_params", w600, w587, w587) -> (w601:refnum<k35>, w599:errorcluster, w593:dbl[])  [unwired: 1 in, 2 out]
                                n327 = Index Array(array=w593, index #1=0, index #2=1, index #3=2) -> (element #1=w596:dbl, element #2=w594:dbl, element #3=w595:dbl)
                                n328 = local write "Px"(w596) -> ()
                                n329 = local write "Py"(w594) -> ()
                                n330 = local write "Phase offset"(w595) -> ()
                              }
                              frame True {
                                n331 = node(w612, w611, "phase_level", w620, w619, w619, w616, w615, w617) -> (w614:refnum<k35>, w613:errorcluster, w618:dbl[][])  [unwired: 4 in, 2 out]
                              }
                            }
                            "Phase" <- w572
                          }
                        }
                      }
                    }
                  }
                }
              }
              n332 = Or(x=w459, y=w451) -> (x .or. y?=w458:bool)
            }
          }
          frame #2 {
            n333 = Wait (ms)(milliseconds to wait=1000) -> ()  [unwired: 1 out]
          }
          frame #3 {
            # "Return to origin postiion"
            n334 = invoke class="StepperMotorChannel" method="SetMoveAbsolutePosition"(reference=w626, "position"=w624) -> (reference out=w632:refnum<k24>, error out=w630:errorcluster)  [unwired: 2 in, 2 out]
            n335 = invoke class="StepperMotorChannel" method="MoveAbsolute"(reference=w632, error in=w630, "waitTimeout"=20000) -> ()  [unwired: 1 in, 4 out]
            n336 = invoke class="StepperMotorChannel" method="SetMoveAbsolutePosition"(reference=w625, "position"=w623) -> (reference out=w629:refnum<k24>, error out=w627:errorcluster)  [unwired: 2 in, 2 out]
            n337 = invoke class="StepperMotorChannel" method="MoveAbsolute"(reference=w629, error in=w627, "waitTimeout"=20000) -> ()  [unwired: 1 in, 4 out]
          }
          frame #4 {
            n338 = One Button Dialog(message="Scan Complete", button name ("OK")="OK") -> ()  [unwired: 1 out]
          }
        }
      }
    }
    n339 = local read "Halt program"() -> (w323:bool)
  }
  n340 = Close Python Session(session in=w25, error in=w24) -> ()  [unwired: 1 out]
  n341 = invoke class="StepperMotorChannel" method="Disconnect"(reference=w23, error in=w22) -> ()  [unwired: 1 in, 3 out]
  n342 = flat-sequence {
    frame #0 {
      n343 = local read "KCubeStepperControl t"() -> (w637:refnum<k24>)
      n344 = local read "SerialNumber t"() -> (w636:string)
      n345 = local read "t Motor Settings"() -> (w635:T2)
      n346 = call "ActionEngine(V2).vi"("ChannelNumber"=4, "Settings"=w635, "SerialNumber"=w636, "KCubeStepperControl"=w637, "Action"=ActionEngineEnum."Close Connection") -> ()  [unwired: 4 in, 2 out]
    }
    frame #1 {
      n347 = local read "KCubeStepperControl t"() -> (w642:refnum<k24>)
      n348 = local read "SerialNumber t"() -> (w643:string)
      n349 = local read "t Motor Settings"() -> (w644:T2)
      n350 = call "ActionEngine(V2).vi"("ChannelNumber"=4, "Settings"=w644, "SerialNumber"=w643, "KCubeStepperControl"=w642, "Action"=ActionEngineEnum."Done") -> ()  [unwired: 4 in, 2 out]
    }
  }
